vi "SP_Position_Set.vi"() -> ()   [LabVIEW 2013]
uses:
  <vilib>/event_ctls.llb/eventvkey.ctl
  Global_Not-Aus.vi
  <vilib>/Utility/file.llb/Write To Spreadsheet File (DBL).vi
  <vilib>/Utility/file.llb/Read From Spreadsheet File (string).vi
  Global_Start_Stop_Einzelschritt.vi
panel:
  in  "Stop Program":bool
  in  "Port for KOSY3":refnum<visa-resource-name>="COM2"
  in  "Port for Powersupply":refnum<visa-resource-name>="COM3"
  in  "Port for Write Head":refnum<visa-resource-name>="COM4"
  in  "Port for ED33":refnum<visa-resource-name>="COM7"
  in  "Port for ED32i":refnum<visa-resource-name>="COM8"
  in  "X,Y,Z Value Limits":T1={"mm Xmin "=0.0, "mm Xmax "=100.0, " mm Ymin "=0.0, "mm Ymax "=267.9, " mm Zmin"=0.0, "mm Zmax "=108.0, "Schritte oder mm Umin (0)"=0.0, "Schritte oder mm Umax (0)"=0.0, "Schritte oder mm Cmin (0)"=0.0, "Schritte oder mm Cmax (0)"=0.0, "Schritte oder mm Amin (0)"=0.0, "Schritte oder mm Amax (0)"=0.0, "Schritte oder mm Bmin (0)"=0.0, "Schritte oder mm Bmax (0)"=0.0}
  out "Error Out":errorcluster caption="error out"
  in  "Error In":errorcluster caption="error in"
  out "Movement":T2={"Axis"=36, "Direction(To/From)"=0, "Speed in mm/s\n (5)[0,025-20]"=5.0, "IV6"=FALSE} {"Direction(To/From)" items=["vom Endschalter weg", "zum Endschalter hin"]; "Speed in mm/s\n (5)[0,025-20]" min=0.025 max=20; "Axis" items=["X-Achse"=36, "Y-Achse"=37, "Z-Achse"=38, "U-Achse"=63]}
  out "Keyboard Press Display":cluster{"Speed(+/-)":i16, "Movement":T3}
  in  "Count":dbl
  in  "Move & Measure":bool
  in  "Clear Sensor Readings":bool
  in  "ED32i Active?":bool
  in  "ED33 Active?":bool
  out "ED33_output":string[][](array[string])
  out "ED32i_output":string[][](array[string])
  out "ED33":i32[](graph)
  out "ED32i":cluster{"Array 4[0]":i32, "Array 4[1]":i32}(graph)
  out "Steps":dbl
  out "Current Sequence":string[](array[string])
  in  "Clear Sequence":bool
  in  "Load Sequence":bool
  out "Sequence":string[][](array[string])
  in  "File  Select":path
  in  "Activate Sequence?":bool
  in  "Tab Control":enum32{"Page 2"}(tab)
  in  "Main Tab":enum32{"Page 1", "Page 2"}(tab)
  in  "Multiple Control":enum32{"Manual Control"}(tab)
  out "P6":dbl[](array[numeric])
  out "P5":dbl[](array[numeric])
  out "P4":dbl[](array[numeric])
  out "P3":dbl[](array[numeric])
  out "P7":dbl[](array[numeric])
  out "P2":dbl[](array[numeric])
  out "P1":dbl[](array[numeric])
  out "P8":dbl[](array[numeric])
  out "P9":dbl[](array[numeric])
  out "P10":dbl[](array[numeric])
  in  "Z axis":enum16{"Up", "Down"}(ring)
  in  "Y axis":enum16{"Forward", "Backward"}(ring)
  in  "X axis":enum16{"Left", "Right"}(ring)
  in  "Move Steps":bool
  in  "Steps(mm)":dbl[](array[numeric]) min=0.0
  in  "Go To":bool
  in  "Position":T4(ring)
  in  "Save":bool
  in  "Reset All":bool
  in  "Reset":bool
  in  "Import":bool
  in  "Export":bool
  in  "File Path":path=path "Y:/01_Projekte/EPN93031_Schreibplatz/8_Konstruktionsunterlagen/8.5_Software/COPY_KOSY Steuerung LabVIEW/1.New_Code_2014_2015/2Pole_strip_Position.txt"
  out "Speed":dbl(knob) scale=0.0..10.0
  out "Operation Done":string="Initialise"
  out "Current Status":string="Initialise"
  out "Moving":bool
  out "Stopped":bool
  in  "Home Position":bool
  out "Current Cordinates":T5 {"Schritte B" format="%#.4g"; "Schritte A" format="%#.4g"; "Schritte C" format="%#.4g"; "Schritte U" format="%#.4g"; "Z axis" format="%#.4g"; "Y axis" format="%#.4g"; "X axis" format="%#.4g"}
  # "Com port info"
  # "Instructions\n                                              Manual Control\n1. Run the program.\n2. Select 'Initialise' to start the program from first \n     or 'Continue' to continue the ongoing process.\n3. Select 'Normal Operation'.\n\nPolestrip Positions\n1. If already positions are already saved, select the corresponding \n    file in 'File Path' and then click 'Import' to get the corresponding\n    positions displayed on the front panel. \n2. Set the 'Speed' using (+/-) for the movement.\n3. Select a position from the dropdown 'Position'and click 'Go To'.\n    Else, \n1. Set the 'Speed' using (+/-) for the movement.\n2. Set the length for movement in 'Steps(mm)'  in corresponding \n    axis and also the direction of travel in the selected axis. \n    Then press 'Move'.\n3. Once desired position is reached, select a position from the \n    dropdown 'Position' and click 'Save'.\n4. Once all positions are saved in front panel, select the file  to be \n     saved in 'File Path' and click 'Export' to save positions to a text file.\n5. Select a position from the dropdown 'Position' and \n    Click 'Reset' to clear individual position.\n6. Click 'Reset All' to clear all positions.\n \nSensor Readings\nContinuous measurement\n1.Activate the sensor to be read from 'Read Sensors' tab.\n2.Set the length for movement in 'Steps(mm)' in corresponding \n    axis and also the direction of travel in the selected axis. \n    Then press 'Move'.\nMove and Measure\n1. Activate the sensor to be read from 'Read Sensors' tab.\n2.Set 'Count' to the number of times to measure.\n2.Set the length for movement in 'Steps(mm)' in corresponding \n    axis and also the direction of travel in the selected axis. \n    Then press 'Move Measure'.\n\n1. Click 'Clear' in 'Read Sensors' tab to clear the sensor readings.\n\n                                          Automatic Execution\n1. Run the program.\n2. Select 'Initialise' to start the program from first \n     or 'Continue' to continue the ongoing process.\n3. Select 'Normal Operation'.\n4. Select the corresponding file in 'File Select' and then click 'Load' \n    to get the corresponding codes in 'Sequence' .\n5. Click 'Clear' to clear sequence.\n6. Click 'Activate Sequence?' to run the automatic execution. \n\n                                                       General\n1. Click 'Stop Program' to stop the running program.\n2. Click 'Home Position' to take the write head to (0,0,0)."
  # "Instructions\n\n1. Set the 'Speed' using (+/-) for the movement.\n2. Arrow keys can be used to move the platform in a particular\n    axis and corresponding direction.\n     First press - move / Second press - stop\n     OR,\n    Set the length for movement in 'Steps(mm)'  in corresponding \n    axis and also the direction of travel in the selected axis. \n    Then press 'Move'.\n3. Once desired position is reached, select a position from the \n    dropdown 'Position' and click 'Save'.\n4. Once all positions are saved in front panel, select the file  to be \n     saved, in 'File Path' and click 'Export' to save positions to a text file.\n5. Select a position from the dropdown 'Position' and \n    Click 'Reset' to clear individual position.\n6. Click 'Reset All' to clear all positions.\n7. Once positions are saved, select the file in 'File Path' and\n     then 'Import' to get the positions displayed ."
  # "Polestrip Positions"
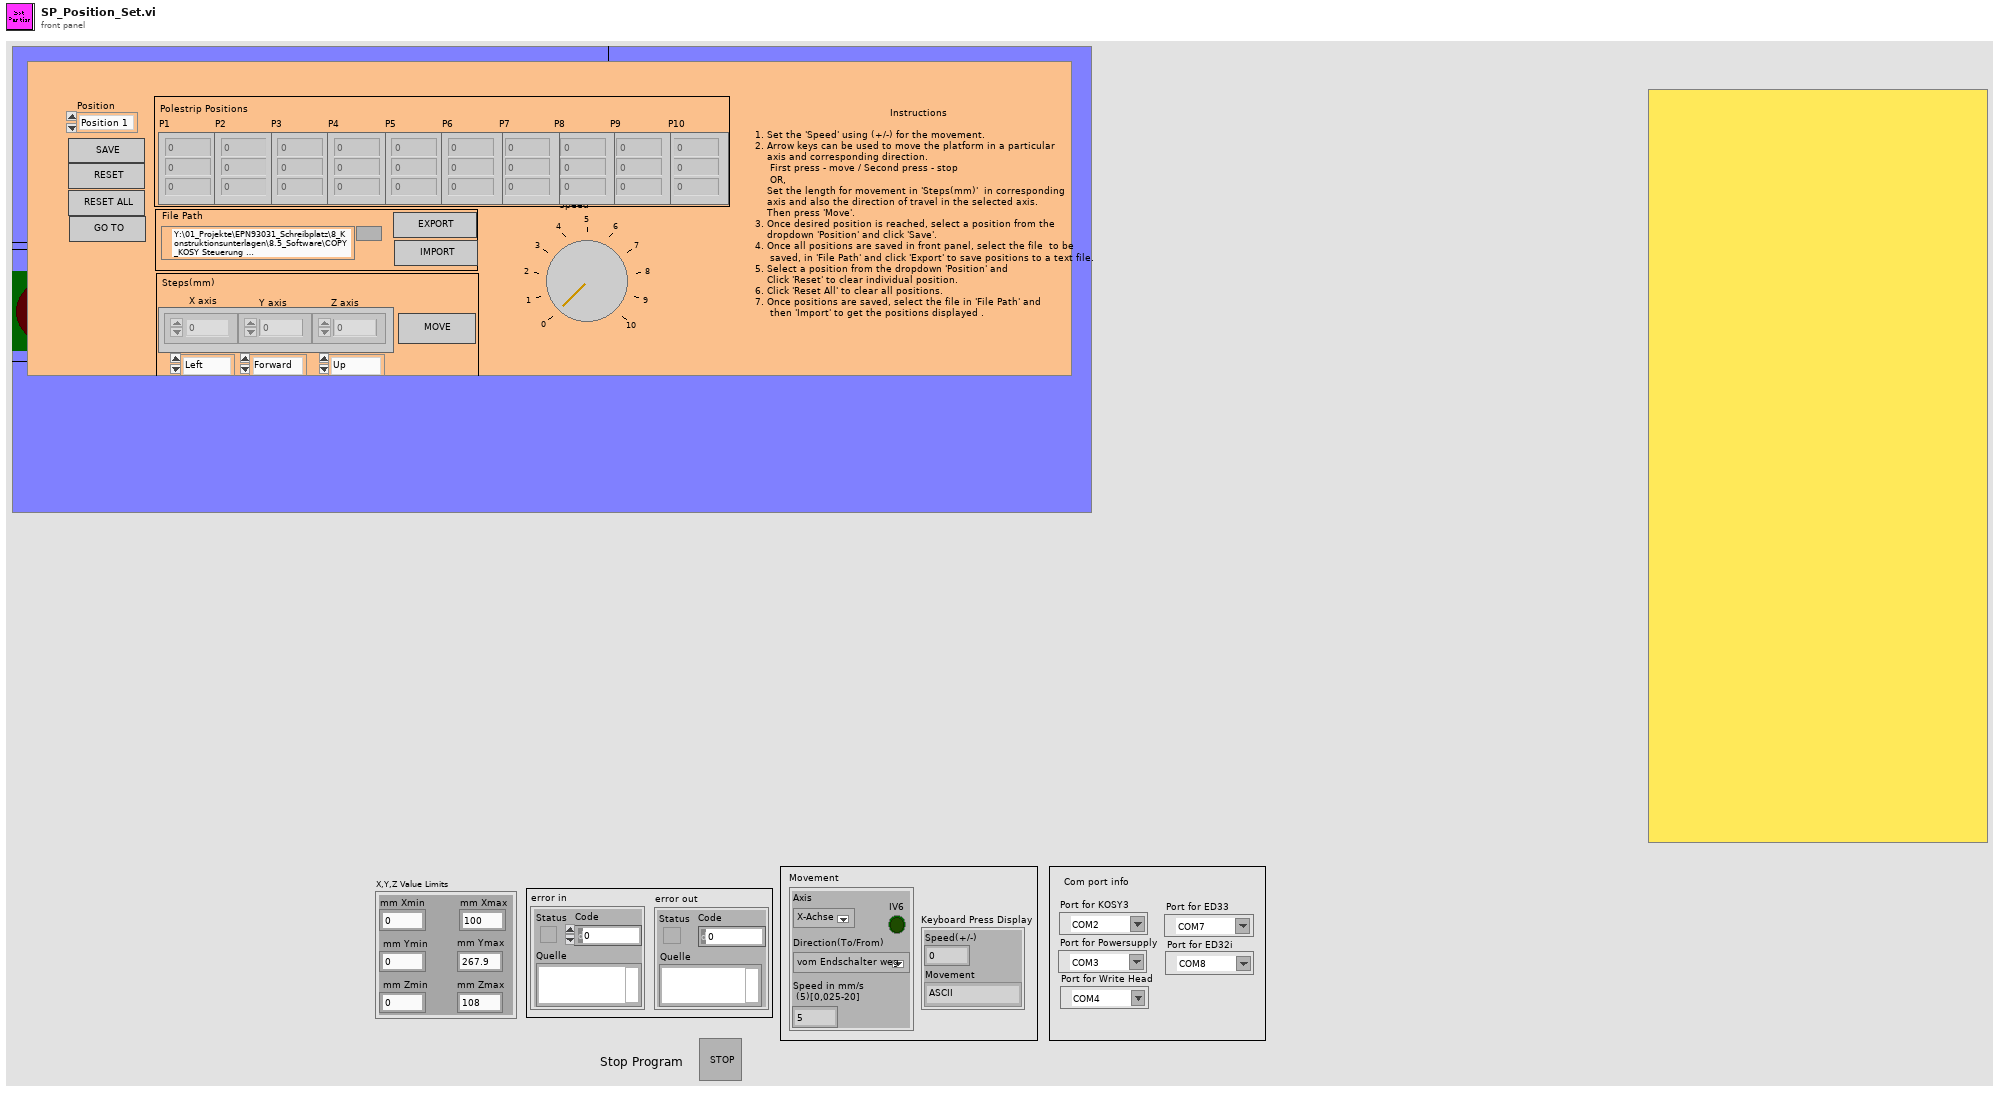
[diagram p1: front panel]
types:
  T1 = cluster{"mm Xmin ":sgl, "mm Xmax ":sgl, " mm Ymin ":sgl, "mm Ymax ":sgl, " mm Zmin":sgl, "mm Zmax ":sgl, "Schritte oder mm Umin (0)":sgl, "Schritte oder mm Umax (0)":sgl, "Schritte oder mm Cmin (0)":sgl, "Schritte oder mm Cmax (0)":sgl, "Schritte oder mm Amin (0)":sgl, "Schritte oder mm Amax (0)":sgl, "Schritte oder mm Bmin (0)":sgl, "Schritte oder mm Bmax (0)":sgl}
  T2 = cluster{"Axis":u8, "Direction(To/From)":u8, "Speed in mm/s\n (5)[0,025-20]":sgl, "IV6":bool}
  T3 = typedef "eventvkey.ctl" = enum16{"ASCII", "Enter", "Return", "Shift", "Ctrl", "Alt", "Cmd", "Opt", "Caps", "NumLock", "Clear", "Break", "Up", "Down", "Left", "Right", "Insert", "Delete", "Home", "End", "PageUp", "PageDown", "Escape", "Help", "Pause", "ScrollLock", "F1", "F2", "F3", "F4", "F5", "F6", "F7", "F8", "F9", "F10", "F11", "F12", "F13", "F14", "F15", "F16", "F17", "F18", "F19", "F20", "F21", "F22", "F23", "F24", "Play", "VolumeUp", "VolumeDown", "Mute", "Two Byte Char"}
  T4 = enum16{"Position 1", "Position 2", "Position 3", "Position 4", "Position 5", "Position 6", "Position 7", "Position 8", "Position 9", "Position 10"}
  T5 = cluster{"X axis":sgl, "Y axis":sgl, "Z axis":sgl, "Schritte U":sgl, "Schritte C":sgl, "Schritte A":sgl, "Schritte B":sgl}
  T6 = cluster{"Geschwindigkeit X in mm/s\n(5) [0,025-15]":sgl, "Geschwindigkeit Y in mm/s\n(5) [0,025-15]":sgl, "Geschwindigkeit Z in mm/s\n(5) [0,025-15]":sgl, "GeschwindigkeitU in mm/s\n(5) [0,025-15]":sgl}
  T7 = cluster{"Schritte X":sgl, "Schritte Y":sgl, "Schritte Z":sgl, "Schritte U":sgl, "Schritte C":sgl, "Schritte A":sgl, "Schritte B":sgl}
  T8 = cluster{"[0]":dbl, "[1]":dbl, "[2]":dbl, "[3]":dbl, "[4]":dbl, "[5]":dbl, "[6]":dbl, "[7]":dbl, "[8]":dbl}
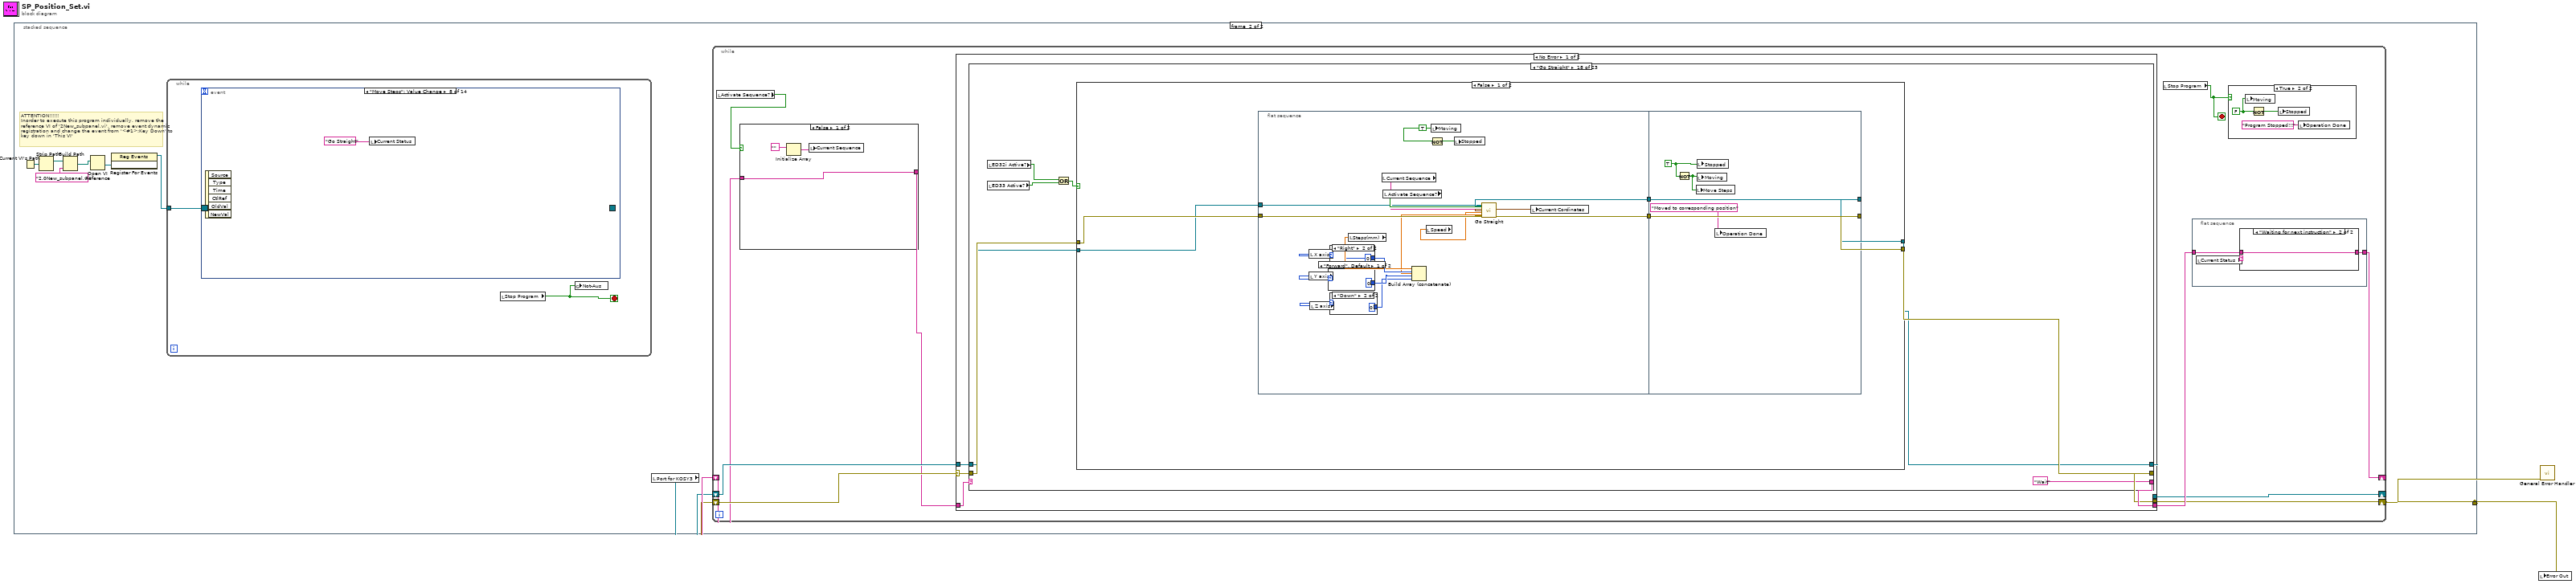
[diagram p0: block diagram]
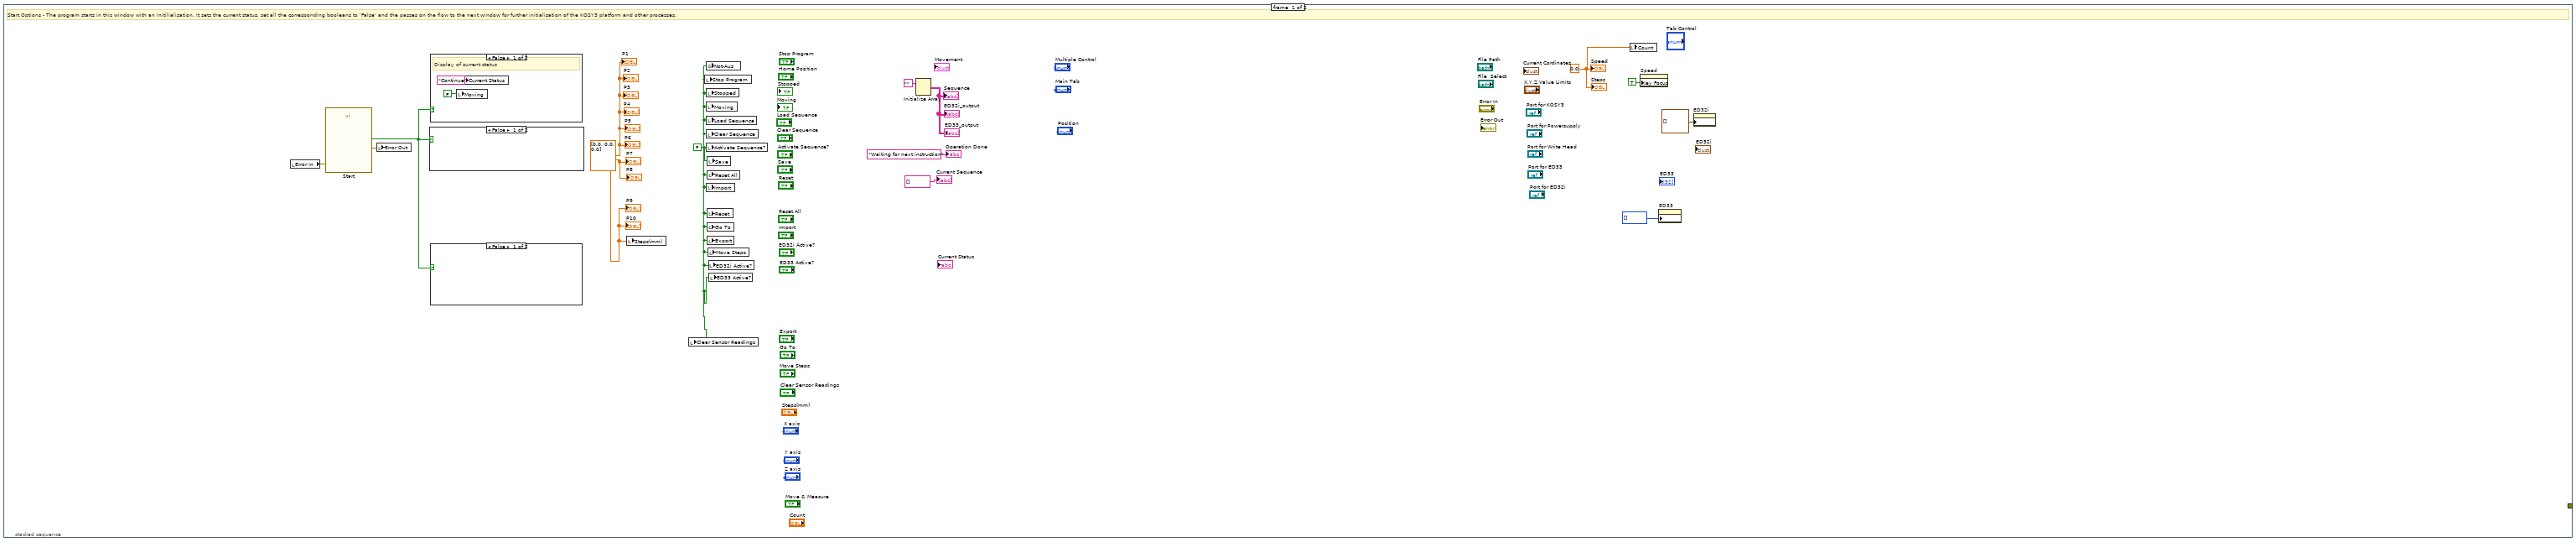
[diagram p2: hidden frame]
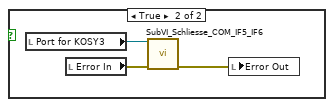
[diagram p3: hidden frame]
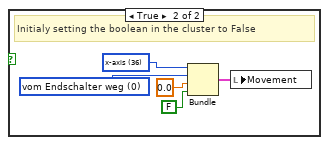
[diagram p4: hidden frame]
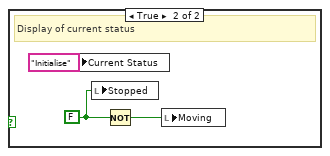
[diagram p5: hidden frame]
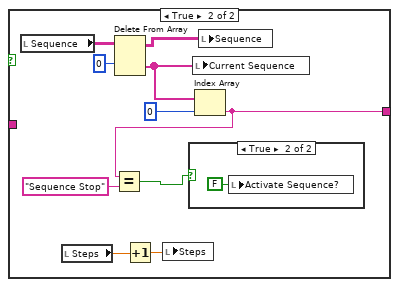
[diagram p6: hidden frame]
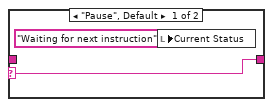
[diagram p9: hidden frame]
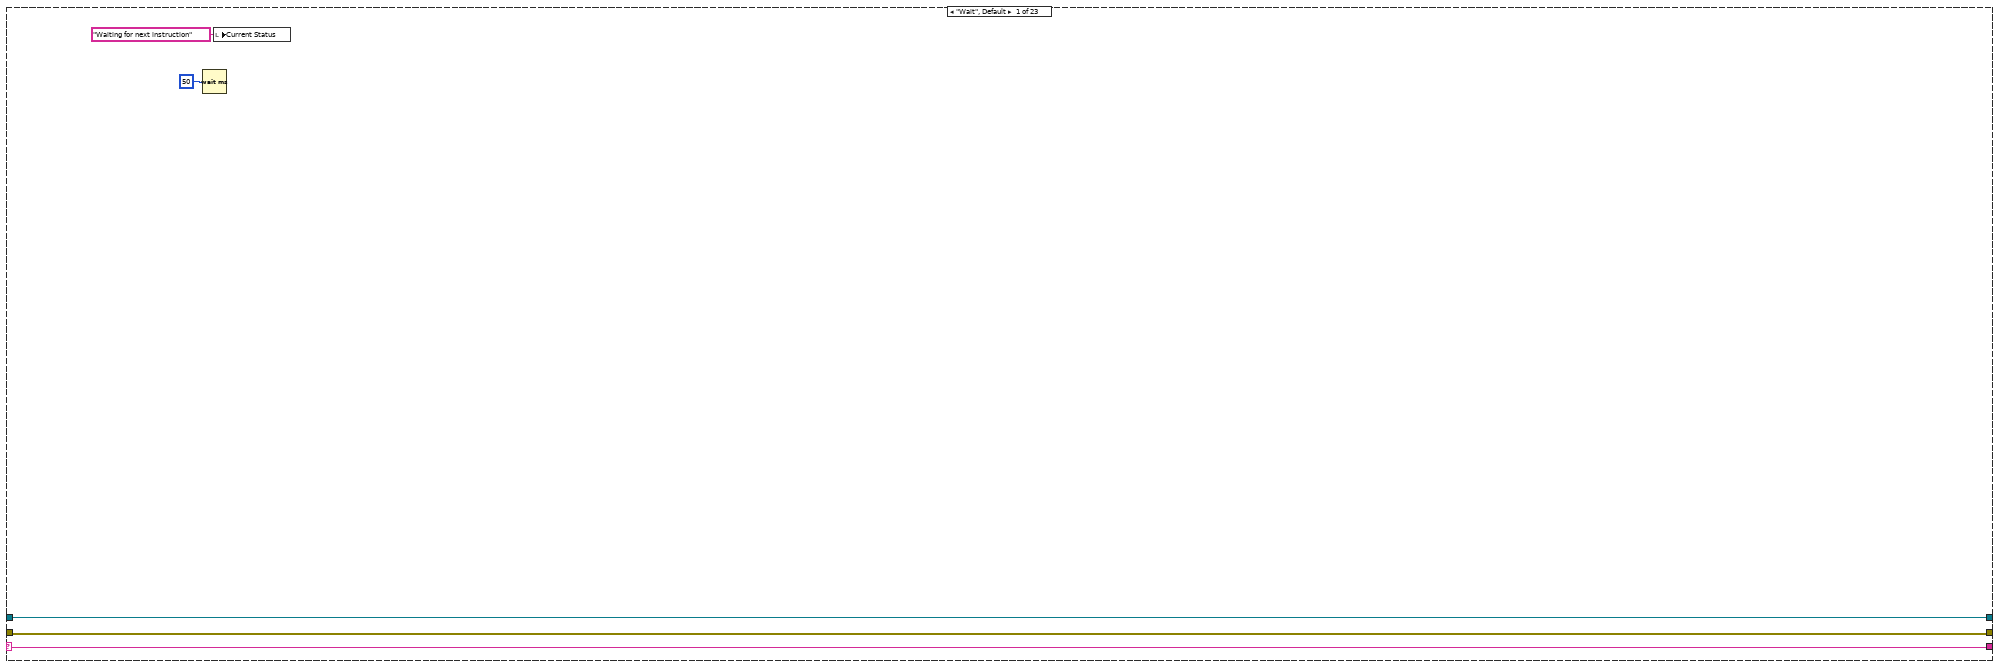
[diagram p10: hidden frame]
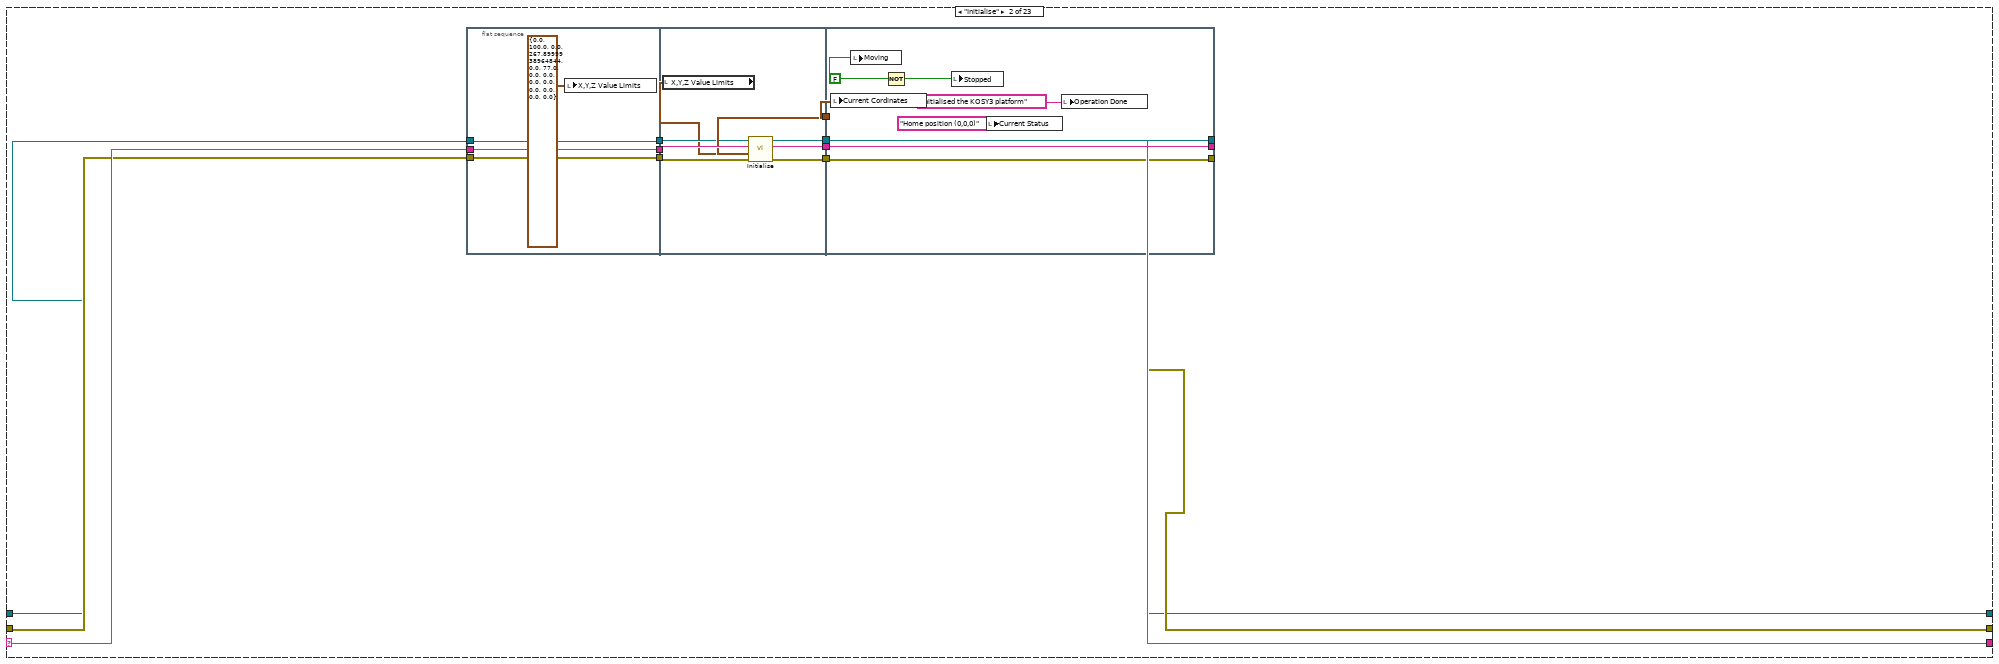
[diagram p11: hidden frame]
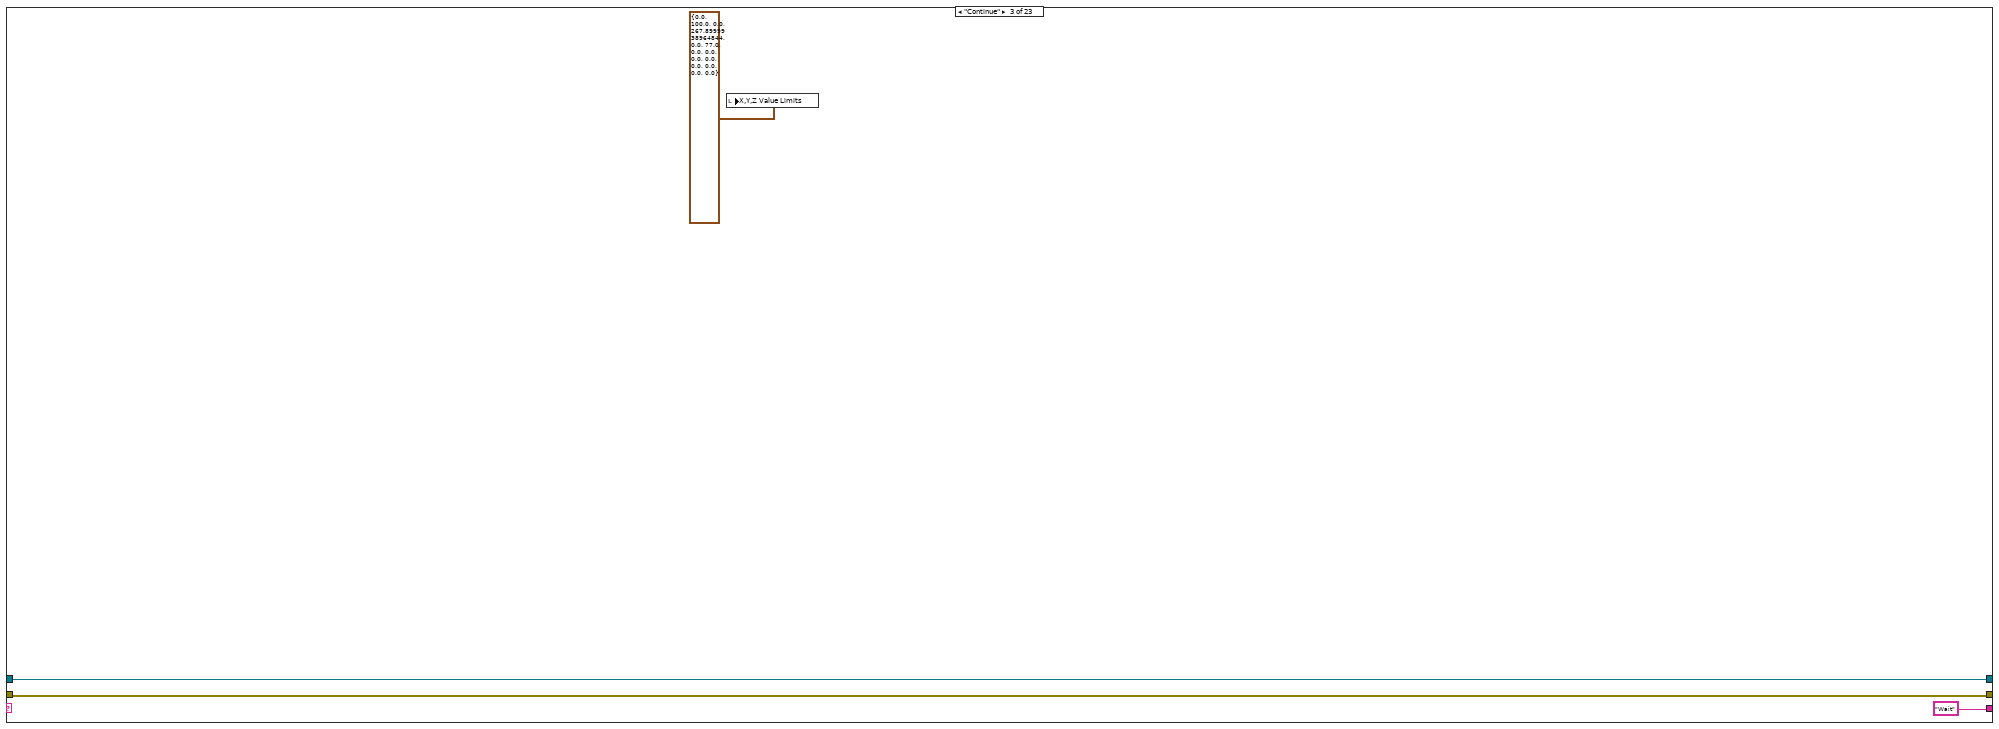
[diagram p12: hidden frame]
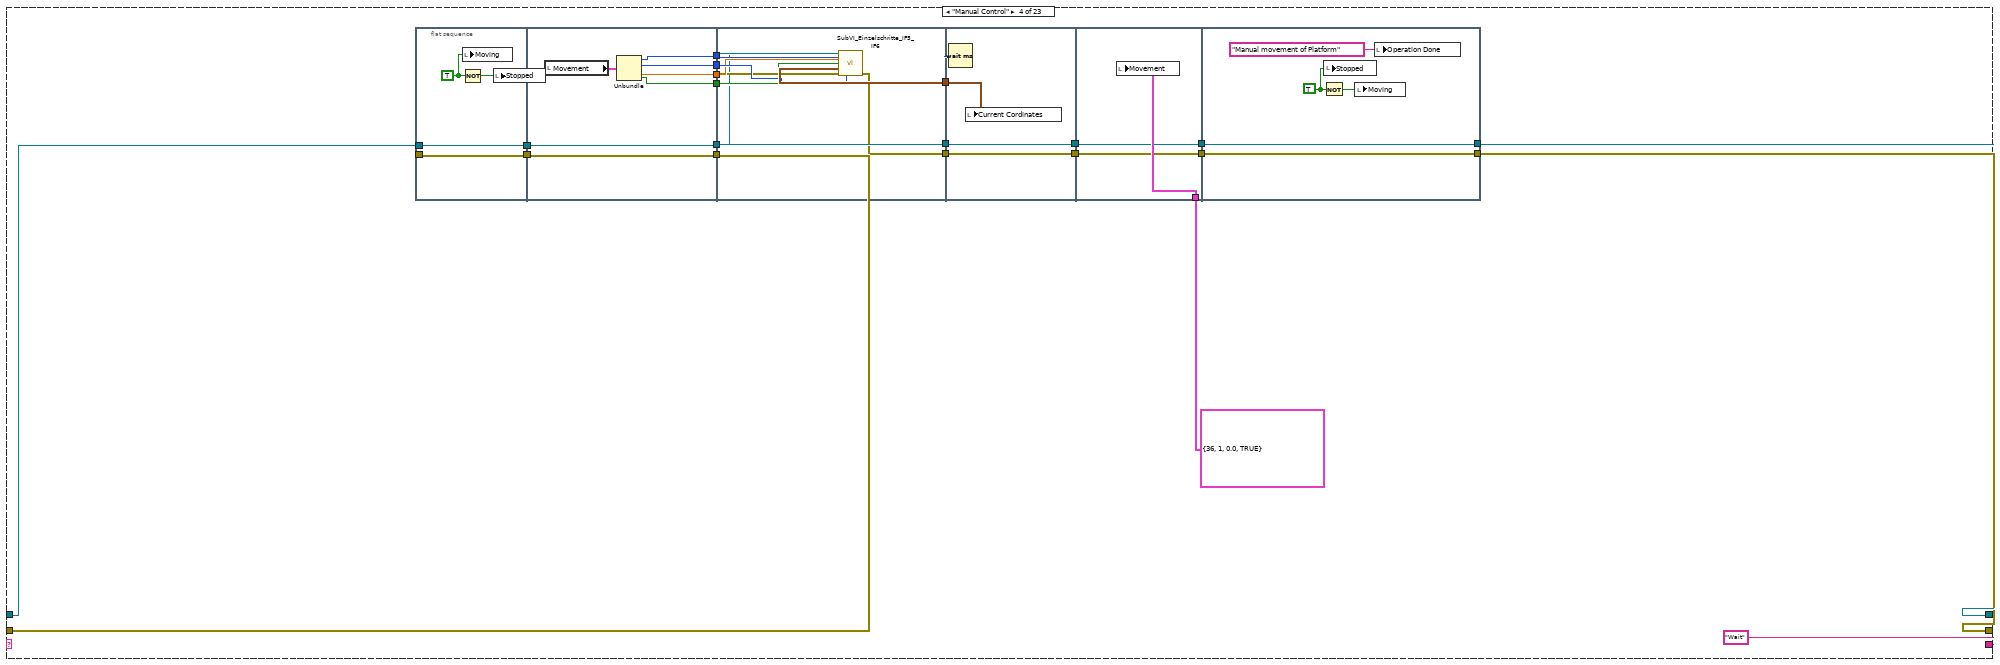
[diagram p13: hidden frame]
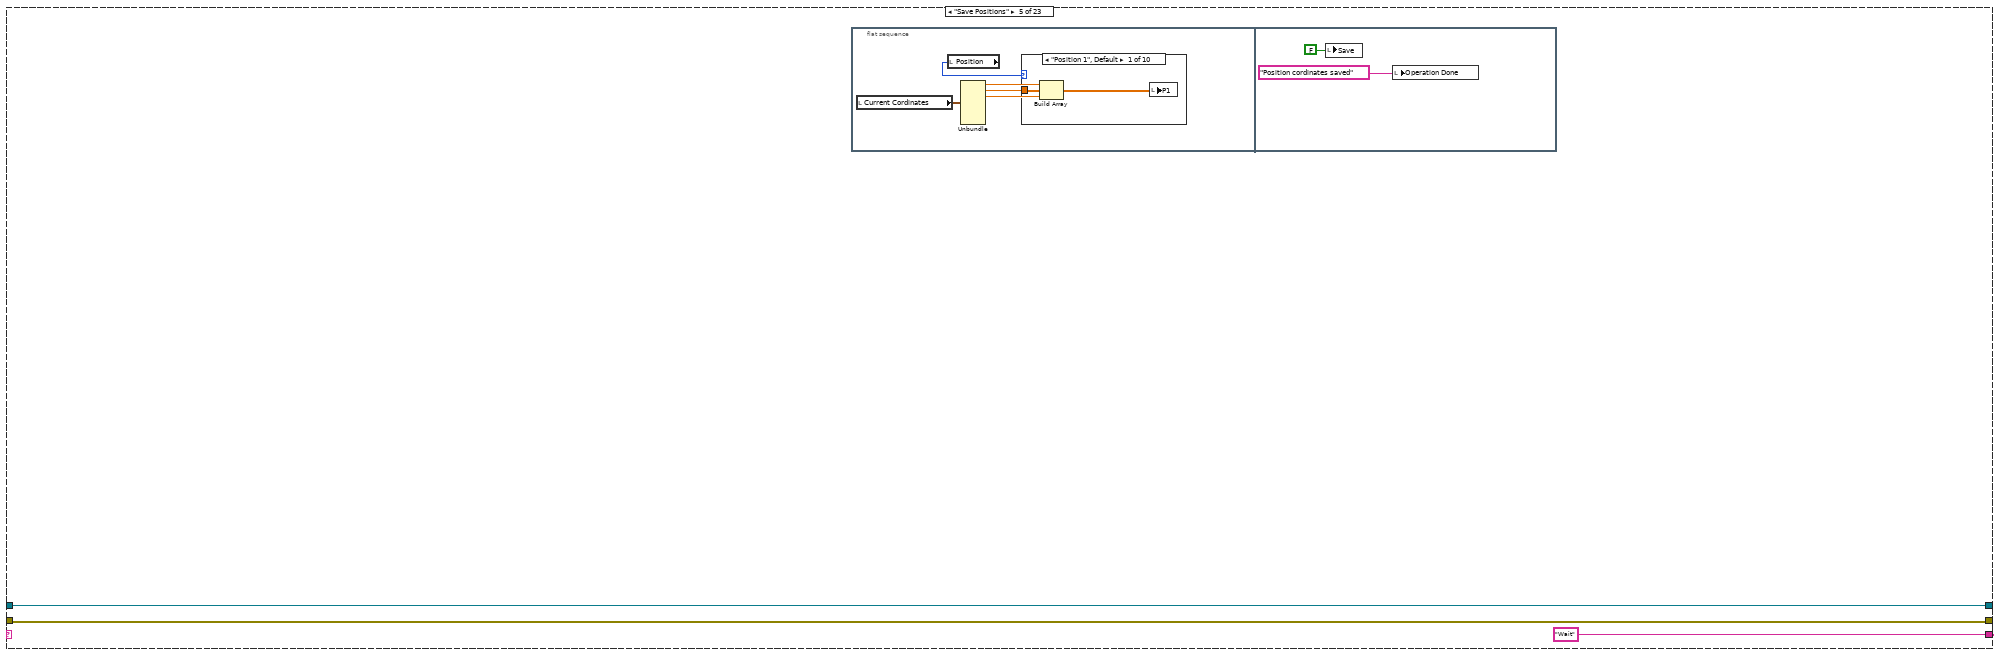
[diagram p14: hidden frame]
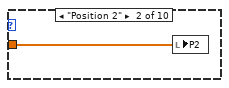
[diagram p15: hidden frame]
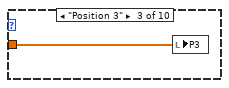
[diagram p16: hidden frame]
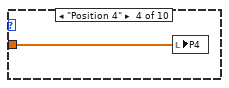
[diagram p17: hidden frame]
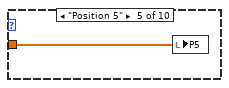
[diagram p18: hidden frame]
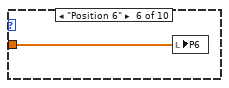
[diagram p19: hidden frame]
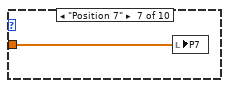
[diagram p20: hidden frame]
diagram:
  n1 = stacked-sequence {
    tunnel: [_ w34] -> w1
    frame #0 {
      w3 = 0.0 ("Speed")
      w4 = dbl[] [0.0, 0.0, 0.0] ("P1")
      w7 = FALSE ("Moving")
      # "Start Options - The program starts in this window with an initilialisation. It sets the current status, set all the corresponding booleans to 'False' and the passes on the flow to the next window for further initialisation of the KOSY3 platform and other processes."
      n2 = local read "Error In"() -> (w14:errorcluster)
      n3 = call "Start"("error in (no error)"=w14) -> ("Initialise"=w12:bool, "error out"=w13:errorcluster)  [unwired: 17 in]
      n4 = local write "Error Out"(w13) -> ()
      n5 = case shown="False" w12 {
        frame False {
        }
        frame True {
          n6 = local read "Port for KOSY3"() -> (w17:refnum<visa-resource-name>)
          n7 = local read "Error In"() -> (w16:errorcluster)
          n8 = call "SubVI_Schliesse_COM_IF5_IF6.vi"("VISA resource name in"=w17, "error in"=w16) -> ("error out"=w15:errorcluster)  [unwired: 13 in]
          n9 = local write "Error Out"(w15) -> ()
        }
      }
      n10 = case shown="False" w12 {
        frame False {
          # "Display of current status"
          n11 = local write "Moving"(FALSE ("Stopped")) -> ()
          n12 = local write "Current Status"("Continue") -> ()
        }
        frame True {
          w25 = FALSE ("Stopped")
          # "Display of current status"
          n13 = local write "Current Status"("Initialise") -> ()
          n14 = local write "Stopped"(w25) -> ()
          n15 = Not(x=w25) -> (.not. x?=w26:bool)
          n16 = local write "Moving"(w26) -> ()
        }
      }
      n17 = case shown="False" w12 {
        frame False {
        }
        frame True {
          w21 = u16 0 items=["vom Endschalter weg", "zum Endschalter hin"]
          w22 = u16 36 items=["x-axis"=36, "y-axis"=37, "z-axis"=38]
          # "Initialy setting the boolean in the cluster to False"
          n18 = Bundle(w22, w21, 0.0, FALSE) -> (w18:cluster{u16, u16, dbl, bool})  [unwired: 1 in]
          n19 = local write "Movement"(w18) -> ()
        }
      }
      n20 = local write "Steps(mm)"(w4) -> ()
      n21 = local write "Clear Sensor Readings"(w7) -> ()
      n22 = local write "Stop Program"(w7) -> ()
      n23 = global write "Global_Not-Aus.vi" "Not-Aus"(w7) -> ()
      n24 = local write "Stopped"(w7) -> ()
      n25 = local write "Moving"(w7) -> ()
      n26 = local write "Load Sequence"(w7) -> ()
      n27 = local write "Clear Sequence"(w7) -> ()
      n28 = local write "Activate Sequence?"(w7) -> ()
      n29 = local write "Import"(w7) -> ()
      n30 = local write "Reset All"(w7) -> ()
      n31 = local write "Reset"(w7) -> ()
      n32 = local write "Go To"(w7) -> ()
      n33 = local write "Export"(w7) -> ()
      n34 = local write "Save"(w7) -> ()
      n35 = local write "Move Steps"(w7) -> ()
      n36 = local write "ED32i Active?"(w7) -> ()
      n37 = local write "ED33 Active?"(w7) -> ()
      n38 = Initialize Array("" ("element")) -> (→"Sequence" →"ED32i_output" →"ED33_output":string[][])  [unwired: 2 in]
      n39 = local write "Count"(w3) -> ()
      n40 = property on="Speed" class="Knob (strict)"("Key Focus"=TRUE) -> ()  [unwired: 2 in, 2 out]
      n41 = property on="ED33" class="WFChart (strict)"("History Data"=i32[] []) -> ()  [unwired: 2 in, 2 out]
      n42 = property on="ED32i" class="WFChart (strict)"("History Data"=cluster{"Array 4[0]":i32, "Array 4[1]":i32}[] []) -> ()  [unwired: 2 in, 2 out]
      "Speed" <- w3
      "P1" <- w4
      "P2" <- w4
      "P3" <- w4
      "P7" <- w4
      "P4" <- w4
      "P5" <- w4
      "P6" <- w4
      "P8" <- w4
      "P9" <- w4
      "P10" <- w4
      "Current Sequence" <- string[] [] ("Current Sequence")
      "Operation Done" <- "Waiting for next instruction" ("Operation Done")
      "Steps" <- w3
    }
    frame #1 {
      # "ATTENTION!!!!!!\nInorder to execute this program individually, remove the reference VI of '2New_subpanel.vi', remove event dynamic registration and change the event from '<#1>:Key Down' to key down in 'This VI'"
      n43 = Current VI's Path() -> (path=w32:path)
      n44 = Strip Path(path=w32) -> (stripped path=w31:path)  [unwired: 1 out]
      n45 = Build Path(base path=w31, name or relative path="2.0New_subpanel.vi") -> (appended path=w29:path)
      n46 = Open VI Reference(vi path=w29) -> (vi reference=w33:refnum<vi>)  [unwired: 5 in, 1 out]
      n47 = register-events(w33) -> (reference out=w28:refnum<event-registration>)  [unwired: 2 in, 1 out]
      n48 = while {
        tunnel: w28 -> [w692]
        stop <- w691 stop-if-true
        n49 = event shown="[7] \"Move Steps\": Value Change" {
          selector: w692 -> [_ w694 _ _ _ _ _ _ _ _ _ _ _ _]
          dyn-events: [_ w694 _ _ _ _ _ _ _ _ _ _ _ _] -> _
          timeout: _ -> [_ _ _ _ _ _ _ _ _ _ _ _ _ _]
          event Timeout {
            n50 = event-data() -> ()  [unwired: 1 in, 2 out]
            n51 = global write "Global_Start_Stop_Einzelschritt.vi" "Boolesch"(FALSE ("Boolesch")) -> ()
          }
          event Key Down {
            # "This window checks for the key press in key board. Upon detection, it would set speed and (or) movement cluster and also updates the status."
            n52 = event-data() -> ("Char"=w695:i16, "VKey"=w697:T3)  [unwired: 1 in, 8 out]
            n53 = Wait (ms)(milliseconds to wait=u32 200) -> ()  [unwired: 1 out]
            n54 = Bundle("Char"=w695, "VKey"=w697) -> (→"Keyboard Press Display":cluster{"Char":i16, "VKey":T3})  [unwired: 1 in]
            n55 = local read "Moving"() -> (w699:bool)
            n56 = case shown="False" w699 {
              tunnel: w697 -> [w705 _]
              tunnel: w695 -> [w707 _]
              frame False {
                n57 = case shown="\"Up\"" w705 {
                  tunnel: [w708 w711 w714 w717 w720 w723 FALSE] -> w704
                  tunnel: [w710 w713 w716 w719 w722 w725 _] -> w702
                  tunnel: [w709 w712 w715 w718 w721 w724 _] -> w701
                  tunnel: TRUE -> [w708 w711 w714 w717 w720 w723 _]
                  frame "Left" {
                    w709 = u16 1 items=["vom Endschalter weg", "zum Endschalter hin"]
                    w710 = u16 36 items=["x-axis"=36, "y-axis"=37, "z-axis"=38]
                    # "Direction control(VKey identifies the directional keys)"
                  }
                  frame "Right" {
                    w712 = u16 0 items=["vom Endschalter weg", "zum Endschalter hin"]
                    w713 = u16 36 items=["x-axis"=36, "y-axis"=37, "z-axis"=38]
                    # "Direction control"
                  }
                  frame "Up" {
                    w715 = u16 1 items=["vom Endschalter weg", "zum Endschalter hin"]
                    w716 = u16 37 items=["x-axis"=36, "y-axis"=37, "z-axis"=38]
                    # "Direction control"
                  }
                  frame "Down" {
                    w718 = u16 0 items=["vom Endschalter weg", "zum Endschalter hin"]
                    w719 = u16 37 items=["x-axis"=36, "y-axis"=37, "z-axis"=38]
                  }
                  frame "PageUp" {
                    w721 = u16 1 items=["vom Endschalter weg", "zum Endschalter hin"]
                    w722 = u16 38 items=["x-axis"=36, "y-axis"=37, "z-axis"=38]
                  }
                  frame "PageDown" {
                    w724 = u16 0 items=["vom Endschalter weg", "zum Endschalter hin"]
                    w725 = u16 38 items=["x-axis"=36, "y-axis"=37, "z-axis"=38]
                  }
                  frame "Return", Default {
                  }
                }
                n58 = local read "Speed"() -> (w700:dbl)
                n59 = call "Speed_set.vi"("Speed"=w700, "Char"=w707) -> ("Speed"=w706:dbl)
                n60 = local write "Speed"(w706) -> ()
                n61 = case shown="True" w704 {
                  tunnel: w706 -> [_ w730]
                  tunnel: w702 -> [_ w729]
                  tunnel: w701 -> [_ w728]
                  frame False {
                  }
                  frame True {
                    n62 = Bundle(w729, w728, "Speed"=w730, TRUE) -> (w727:cluster{u16, u16, "Speed":dbl, bool})  [unwired: 1 in]
                    n63 = local write "Movement"(w727) -> ()
                    n64 = local write "Current Status"("Manual Control" ("Status")) -> ()
                  }
                }
              }
              frame True {
                n65 = global write "Global_Start_Stop_Einzelschritt.vi" "Boolesch"(TRUE) -> ()
                n66 = local write "Moving"(FALSE) -> ()
              }
            }
          }
          event "Home Position": Value Change {
            # "This window corresponds to the 'Home position' button on the Front Panel. Pressing the button will take KOSY3 paltform to the home position (0,0,0)"
            n67 = event-data() -> ()  [unwired: 1 in, 6 out]
            n68 = local write "Current Status"("Home Position" ("Status")) -> ()
          }
          event "Save": Value Change {
            # "When the 'SAVE' button in the Front Panel is pressed, it would save the current cordinates of the KOSY3 platform to the selected position."
            n69 = event-data() -> ()  [unwired: 1 in, 6 out]
            n70 = local write "Current Status"("Save Positions" ("Status")) -> ()
          }
          event "Reset": Value Change {
            # "When 'RESET' in the Front Panel is pressed, it resets the cordinates in the selected position to (0,0,0)"
            n71 = event-data() -> ()  [unwired: 1 in, 6 out]
            n72 = local write "Current Status"("Reset Position" ("Status")) -> ()
          }
          event "Reset All": Value Change {
            # "When 'RESET ALL' in the Front Panel is pressed, it resets the cordinates in all positions to (0,0,0)"
            n73 = event-data() -> ()  [unwired: 1 in, 6 out]
            n74 = local write "Current Status"("Reset All" ("Status")) -> ()
          }
          event "Go To": Value Change {
            n75 = event-data() -> ()  [unwired: 1 in, 6 out]
            n76 = local write "Current Status"("Go Position" ("Status")) -> ()
          }
          event "Move Steps": Value Change {
            n77 = event-data() -> ()  [unwired: 1 in, 6 out]
            n78 = local write "Current Status"("Go Straight" ("Status")) -> ()
          }
          event "Move & Measure": Value Change {
            n79 = event-data() -> ()  [unwired: 1 in, 6 out]
            n80 = local write "Current Status"("Move & Measure" ("Status")) -> ()
          }
          event "Import": Value Change {
            n81 = event-data() -> ()  [unwired: 1 in, 6 out]
            n82 = local write "Current Status"("Import Cordinates" ("Status")) -> ()
          }
          event "Export": Value Change {
            n83 = event-data() -> ()  [unwired: 1 in, 6 out]
            n84 = local write "Current Status"("Export Cordinates" ("Status")) -> ()
          }
          event "Load Sequence": Value Change {
            n85 = event-data() -> ()  [unwired: 1 in, 6 out]
            n86 = local write "Current Status"("Load Sequence" ("Status")) -> ()
          }
          event "Clear Sequence": Value Change {
            n87 = event-data() -> ()  [unwired: 1 in, 6 out]
            n88 = local write "Current Status"("Clear Sequence" ("Status")) -> ()
          }
          event "Clear Sensor Readings": Value Change {
            n89 = event-data() -> ()  [unwired: 1 in, 6 out]
            n90 = local write "Current Status"("Clear SensorReadings" ("Status")) -> ()
          }
        }
        n91 = local read "Stop Program"() -> (w691:bool)
        n92 = global write "Global_Not-Aus.vi" "Not-Aus"(w691) -> ()
      }
      n93 = local read "Port for KOSY3"() -> (w35:refnum<visa-resource-name>)
      n94 = local read "Current Status"() -> (w37:string)
      n95 = local read "Error In"() -> (w36:errorcluster)
      n96 = while {
        shift-right: [w42] -> w34
        shift-left: w36 -> [w47]
        shift-right: [w43] -> _
        shift-left: w35 -> [w44]
        shift-right: [w45] -> _
        shift-left: w37 -> [w41]
        stop <- w38 stop-if-true
        n97 = local read "Activate Sequence?"() -> (w39:bool)
        n98 = case shown="False" w39 {
          tunnel: w41 -> [w50 _]
          tunnel: [w50 w55] -> w40
          frame False {
            n99 = Initialize Array("") -> (w48:string[])  [unwired: 1 in]
            n100 = local write "Current Sequence"(w48) -> ()
          }
          frame True {
            n101 = local read "Sequence"() -> (w60:string[][])
            n102 = local read "Steps"() -> (w52:dbl)
            n103 = Delete From Array(array=w60, index (row)=0) -> (deleted portion=w57:string[], array with subset deleted=w58:string[][])  [unwired: 2 in]
            n104 = Increment(x=w52) -> (x+1=w51:dbl)
            n105 = local write "Steps"(w51) -> ()
            n106 = local write "Current Sequence"(w57) -> ()
            n107 = Index Array(array=w57, index=0) -> (element=w55:string)
            n108 = Equal?(x=w55, y="Sequence Stop") -> (x = y?=w53:bool)
            n109 = case shown="True" w53 {
              frame False {
              }
              frame True {
                n110 = local write "Activate Sequence?"(FALSE ("Activate Sequence?")) -> ()
              }
            }
            n111 = local write "Sequence"(w58) -> ()
          }
        }
        n112 = case shown="No Error" w47 {
          selector: w47 -> [w73 w686]
          tunnel: w40 -> [w76 _]
          tunnel: [w75 "Error" ("String 2")] -> w46
          tunnel: w44 -> [w74 w687]
          tunnel: [w71 w687] -> w43
          tunnel: [w72 w686] -> w42
          frame No Error {
            n113 = case shown="\"Go Straight\"" w76 {
              selector: w76 -> [w80 w94 _ _ _ _ _ _ _ _ _ _ _ _ _ _ _ _ _ _ _ _ _]
              tunnel: [w80 w91 "Wait" ("String 2") "Wait" "Wait" ("String 2") "Wait" ("String 2") "Wait" ("String 2") "Wait" ("String 2") "Wait" ("String 2") "Wait" ("String 2") "Wait" ("String 2") "Wait" ("String 2") "Wait" ("String 2") "Wait" ("String 2") "Wait" ("String 2") "Wait" ("String 2") "Wait" ("String 2") "Wait" ("String 2") "Wait" ("String 2") "Wait" ("String 2") "Wait" ("String 2") "Wait" ("String 2") "Wait" ("String 2")] -> w75
              tunnel: w74 -> [w77 w89 w117 w127 w173 w194 w211 w221 w253 w269 w308 w331 w338 w347 w356 w365 w379 w414 w536 w565 w573 w671 w678]
              tunnel: w73 -> [w78 w90 w115 w130 w172 w193 w210 w220 w254 w270 w310 w332 w339 w346 w357 w364 w380 w415 w534 w564 w574 w670 w680]
              tunnel: [w78 w87 w115 w122 w172 w193 w210 w218 w254 w270 w305 w332 w339 w346 w357 w364 w381 w413 w534 w564 w574 w670 w679] -> w72
              tunnel: [w77 w85 w117 w126 w173 w194 w211 w219 w253 w269 w307 w331 w338 w347 w356 w365 w382 w412 w536 w565 w572 w671 w678] -> w71
              frame "Wait", Default {
                n114 = Wait (ms)(milliseconds to wait=50) -> ()  [unwired: 1 out]
                n115 = local write "Current Status"("Waiting for next instruction" ("Status")) -> ()
              }
              frame "Initialise" {
                n116 = flat-sequence {
                  tunnel: w89 -> [w96]
                  tunnel: w90 -> [w97]
                  tunnel: w94 -> [w98]
                  tunnel: [w98] -> w84
                  tunnel: [w97] -> w83
                  tunnel: [w96] -> w82
                  tunnel: [w105] -> w93
                  tunnel: [w104] -> w92
                  tunnel: [w101] -> w88
                  tunnel: [w100] -> w86
                  tunnel: w84 -> [w106]
                  tunnel: w83 -> [w103]
                  tunnel: w82 -> [w102]
                  tunnel: w93 -> [w111]
                  tunnel: w92 -> [w110]
                  tunnel: [w110] -> w91
                  tunnel: [w108] -> w85
                  tunnel: w88 -> [w108]
                  tunnel: [w107] -> w87
                  tunnel: w86 -> [w107]
                  frame #0 {
                    n117 = local write "X,Y,Z Value Limits"(T1 {"mm Xmin "=0.0, "mm Xmax "=100.0, " mm Ymin "=0.0, "mm Ymax "=267.9, " mm Zmin"=0.0, "mm Zmax "=77.0, "Schritte oder mm Umin (0)"=0.0, "Schritte oder mm Umax (0)"=0.0, "Schritte oder mm Cmin (0)"=0.0, "Schritte oder mm Cmax (0)"=0.0, "Schritte oder mm Amin (0)"=0.0, "Schritte oder mm Amax (0)"=0.0, "Schritte oder mm Bmin (0)"=0.0, "Schritte oder mm Bmax (0)"=0.0} ("X,Y,Z Value Limits")) -> ()
                  }
                  frame #1 {
                    n118 = local read "X,Y,Z Value Limits"() -> (w99:T1)
                    n119 = call "Initialise.vi"("error IO"=w103, "X,Y,Z values"=w99, "String"=w106, "Port for KOSY3"=w102) -> ("Fehler (Ausgang)"=w100:errorcluster, "Cordinates of the  KOSY3 Platform"=w105:T7, "String 2"=w104:string, "VISA-Referenz (Ausgang)"=w101:refnum<visa-resource-name>)
                  }
                  frame #2 {
                    w112 = FALSE ("Stopped")
                    n120 = local write "Current Cordinates"(w111) -> ()
                    n121 = local write "Moving"(w112) -> ()
                    n122 = Not(x=w112) -> (.not. x?=w113:bool)
                    n123 = local write "Stopped"(w113) -> ()
                    n124 = local write "Current Status"("Home position (0,0,0)" ("Status")) -> ()
                    n125 = local write "Operation Done"("Initialised the KOSY3 platform" ("Operation Done")) -> ()
                  }
                }
              }
              frame "Continue" {
                n126 = local write "X,Y,Z Value Limits"(T1 {"mm Xmin "=0.0, "mm Xmax "=100.0, " mm Ymin "=0.0, "mm Ymax "=267.9, " mm Zmin"=0.0, "mm Zmax "=77.0, "Schritte oder mm Umin (0)"=0.0, "Schritte oder mm Umax (0)"=0.0, "Schritte oder mm Cmin (0)"=0.0, "Schritte oder mm Cmax (0)"=0.0, "Schritte oder mm Amin (0)"=0.0, "Schritte oder mm Amax (0)"=0.0, "Schritte oder mm Bmin (0)"=0.0, "Schritte oder mm Bmax (0)"=0.0} ("X,Y,Z Value Limits")) -> ()
              }
              frame "Manual Control" {
                n127 = flat-sequence {
                  tunnel: [w141] -> w131
                  tunnel: w130 -> [w141]
                  tunnel: [w140] -> w128
                  tunnel: w127 -> [w140]
                  tunnel: [w149] -> w138
                  tunnel: [w148] -> w137
                  tunnel: [w147] -> w136
                  tunnel: [w146] -> w135
                  tunnel: [w145] -> w132
                  tunnel: w131 -> [w145]
                  tunnel: [w144] -> w129
                  tunnel: w128 -> [w144]
                  tunnel: [w159] -> w134
                  tunnel: w138 -> [w158]
                  tunnel: w137 -> [w157]
                  tunnel: w136 -> [w156]
                  tunnel: w135 -> [w155]
                  tunnel: w132 -> [w154]
                  tunnel: w129 -> [w151]
                  tunnel: [w153] -> w123
                  tunnel: [w152] -> w119
                  tunnel: w134 -> [w162]
                  tunnel: [w161] -> w124
                  tunnel: w123 -> [w161]
                  tunnel: [w160] -> w120
                  tunnel: w119 -> [w160]
                  tunnel: cluster{u16, u16, dbl, bool} {36, 1, 0.0, TRUE} -> [w166]
                  tunnel: [w165] -> w125
                  tunnel: w124 -> [w165]
                  tunnel: [w164] -> w121
                  tunnel: w120 -> [w164]
                  tunnel: [w168] -> w126
                  tunnel: w125 -> [w168]
                  tunnel: [w167] -> w122
                  tunnel: w121 -> [w167]
                  frame #0 {
                    w142 = TRUE ("Moving")
                    n128 = Not(x=w142) -> (.not. x?=w143:bool)
                    n129 = local write "Moving"(w142) -> ()
                    n130 = local write "Stopped"(w143) -> ()
                  }
                  frame #1 {
                    n131 = local read "Movement"() -> (w150:T2)
                    n132 = Unbundle(w150) -> ("Axis"=w149:u8, "Direction(To/From)"=w148:u8, "Speed in mm/s\n (5)[0,025-20]"=w147:sgl, "IV6"=w146:bool)
                  }
                  frame #2 {
                    n133 = call <userlib>:"SubVI_Einzelschritte_IF5_IF6.vi"("VISA resource name in"=w151, "Achsen-Wahl (X)"=w158, "Geschwindigkeit\nin mm/s (5)[0,025-20]"=w156, "IF5=F/IF6=T\n(IF6=T) in"=w155, "error in"=w154, "Richtung (vEw)"=w157) -> ("VISA resource name out"=w153:refnum<visa-resource-name>, "Koordinaten IF6"=w159:T7, "error out"=w152:errorcluster)  [unwired: 3 in, 4 out]
                  }
                  frame #3 {
                    n134 = Wait (ms)(milliseconds to wait=u32 100) -> ()  [unwired: 1 out]
                    n135 = local write "Current Cordinates"(w162) -> ()
                  }
                  frame #4 {
                    n136 = local write "Movement"(w166) -> ()
                  }
                  frame #5 {
                    w171 = TRUE ("Moving")
                    n137 = Not(x=w171) -> (.not. x?=w170:bool)
                    n138 = local write "Stopped"(w171) -> ()
                    n139 = local write "Moving"(w170) -> ()
                    n140 = local write "Operation Done"("Manual movement of Platform" ("Status")) -> ()
                  }
                }
              }
              frame "Save Positions" {
                n141 = flat-sequence {
                  frame #0 {
                    n142 = local read "Current Cordinates"() -> (w178:T5)
                    n143 = local read "Position"() -> (w180:T4)
                    n144 = Unbundle(w178) -> ("X axis"=w175:sgl, "Y axis"=w176:sgl, "Z axis"=w177:sgl)  [unwired: 4 out]
                    n145 = Build Array(w175, w176, w177) -> (w179:sgl[])
                    n146 = case shown="\"Position 1\", Default" w180 {
                      tunnel: w179 -> [w181 w182 w183 w184 w185 w186 w187 w188 w189 w190]
                      frame "Position 1", Default {
                        n147 = local write "P1"(w181) -> ()
                      }
                      frame "Position 2" {
                        n148 = local write "P2"(w182) -> ()
                      }
                      frame "Position 3" {
                        n149 = local write "P3"(w183) -> ()
                      }
                      frame "Position 4" {
                        n150 = local write "P4"(w184) -> ()
                      }
                      frame "Position 5" {
                        n151 = local write "P5"(w185) -> ()
                      }
                      frame "Position 6" {
                        n152 = local write "P6"(w186) -> ()
                      }
                      frame "Position 7" {
                        n153 = local write "P7"(w187) -> ()
                      }
                      frame "Position 8" {
                        n154 = local write "P8"(w188) -> ()
                      }
                      frame "Position 9" {
                        n155 = local write "P9"(w189) -> ()
                      }
                      frame "Position 10" {
                        n156 = local write "P10"(w190) -> ()
                      }
                    }
                  }
                  frame #1 {
                    n157 = local write "Save"(FALSE ("Save Button")) -> ()
                    n158 = local write "Operation Done"("Position cordinates saved" ("Operation Done")) -> ()
                  }
                }
              }
              frame "Reset Position" {
                n159 = flat-sequence {
                  frame #0 {
                    n160 = local read "Position"() -> (w196:T4)
                    n161 = case shown="\"Position 10\"" w196 {
                      tunnel: dbl[] [0.0, 0.0, 0.0] ("P1") -> [w198 w199 w200 w201 w202 w203 w204 w205 w206 w207]
                      frame "Position 1", Default {
                        n162 = local write "P1"(w198) -> ()
                      }
                      frame "Position 2" {
                        n163 = local write "P2"(w199) -> ()
                      }
                      frame "Position 3" {
                        n164 = local write "P3"(w200) -> ()
                      }
                      frame "Position 4" {
                        n165 = local write "P4"(w201) -> ()
                      }
                      frame "Position 5" {
                        n166 = local write "P5"(w202) -> ()
                      }
                      frame "Position 6" {
                        n167 = local write "P6"(w203) -> ()
                      }
                      frame "Position 7" {
                        n168 = local write "P7"(w204) -> ()
                      }
                      frame "Position 8" {
                        n169 = local write "P8"(w205) -> ()
                      }
                      frame "Position 9" {
                        n170 = local write "P9"(w206) -> ()
                      }
                      frame "Position 10" {
                        n171 = local write "P10"(w207) -> ()
                      }
                    }
                  }
                  frame #1 {
                    n172 = local write "Reset"(FALSE ("Reset")) -> ()
                    n173 = local write "Operation Done"("The selected position is reset" ("Operation Done")) -> ()
                  }
                }
              }
              frame "Reset All" {
                n174 = flat-sequence {
                  frame #0 {
                    w213 = dbl[] [0.0, 0.0, 0.0] ("P1")
                    n175 = local write "P1"(w213) -> ()
                    n176 = local write "P2"(w213) -> ()
                    n177 = local write "P3"(w213) -> ()
                    n178 = local write "P4"(w213) -> ()
                    n179 = local write "P5"(w213) -> ()
                    n180 = local write "P6"(w213) -> ()
                    n181 = local write "P7"(w213) -> ()
                    n182 = local write "P8"(w213) -> ()
                    n183 = local write "P9"(w213) -> ()
                    n184 = local write "P10"(w213) -> ()
                    n185 = local write "Steps(mm)"(w213) -> ()
                  }
                  frame #1 {
                    n186 = local write "Reset All"(FALSE ("Reset all Positions")) -> ()
                    n187 = local write "Operation Done"("Reset all positions" ("Operation Done")) -> ()
                  }
                }
              }
              frame "Go Position" {
                n188 = flat-sequence {
                  tunnel: [w226] -> w217
                  tunnel: [w225] -> w216
                  tunnel: w221 -> [w228]
                  tunnel: w220 -> [w227]
                  tunnel: [w251] -> w218
                  tunnel: [w252] -> w219
                  tunnel: w217 -> [w252]
                  tunnel: w216 -> [w251]
                  frame #0 {
                    w224 = TRUE ("Moving")
                    n189 = local write "Moving"(w224) -> ()
                    n190 = local read "Position"() -> (w236:T4)
                    n191 = case shown="\"Position 10\"" w236 {
                      tunnel: [w237 w238 w239 w240 w241 w242 w243 w244 w245 w246] -> w234
                      frame "Position 1", Default {
                        n192 = local read "P1"() -> (w237:dbl[])
                      }
                      frame "Position 2" {
                        n193 = local read "P2"() -> (w238:dbl[])
                      }
                      frame "Position 3" {
                        n194 = local read "P3"() -> (w239:dbl[])
                      }
                      frame "Position 4" {
                        n195 = local read "P4"() -> (w240:dbl[])
                      }
                      frame "Position 5" {
                        n196 = local read "P5"() -> (w241:dbl[])
                      }
                      frame "Position 6" {
                        n197 = local read "P6"() -> (w242:dbl[])
                      }
                      frame "Position 7" {
                        n198 = local read "P7"() -> (w243:dbl[])
                      }
                      frame "Position 8" {
                        n199 = local read "P8"() -> (w244:dbl[])
                      }
                      frame "Position 9" {
                        n200 = local read "P9"() -> (w245:dbl[])
                      }
                      frame "Position 10" {
                        n201 = local read "P10"() -> (w246:dbl[])
                      }
                    }
                    n202 = Not(x=w224) -> (.not. x?=w223:bool)
                    n203 = local write "Stopped"(w223) -> ()
                    n204 = local read "Speed"() -> (w230:dbl)
                    n205 = local read "Current Cordinates"() -> (w233:T5)
                    n206 = Bundle(0, "Speed"=w230, 0) -> (w229:cluster{i32, "Speed":dbl, i32})  [unwired: 1 in]
                    n207 = call <userlib>:"SubVI_Punkt_anfahren_IF5_IF6.vi"("Angehängtes Array"=w234, "error in"=w227, "Koordinaten in IF6"=w233, "Geschwindigkeiten"=w229, "VISA resource name in"=w228) -> ("error out"=w225:errorcluster, "Koordinaten out IF6"=w235:T7, "VISA resource name in 2"=w226:refnum<visa-resource-name>)  [unwired: 1 in]
                    n208 = local write "Current Cordinates"(w235) -> ()
                  }
                  frame #1 {
                    w247 = TRUE ("Moving")
                    n209 = local write "Go To"(FALSE ("Go To")) -> ()
                    n210 = local write "Stopped"(w247) -> ()
                    n211 = Not(x=w247) -> (.not. x?=w248:bool)
                    n212 = local write "Moving"(w248) -> ()
                    n213 = local write "Operation Done"("Go to the selected position" ("Operation Done")) -> ()
                  }
                }
              }
              frame "Import Cordinates" {
                n214 = flat-sequence {
                  frame #0 {
                    n215 = local read "File Path"() -> (w266:path)
                    n216 = call "Dekoder Batch Speicher.vi"("Batchfeld Speicher"=w266) -> ("P9"=w256:dbl[], "P10"=w257:dbl[], "P1"=w258:dbl[], "P2"=w259:dbl[], "P8"=w260:dbl[], "P3"=w261:dbl[], "P4"=w262:dbl[], "P7"=w265:dbl[], "P6"=w263:dbl[], "P5"=w264:dbl[])  [unwired: 5 in]
                    n217 = local write "P9"(w256) -> ()
                    n218 = local write "P10"(w257) -> ()
                    n219 = local write "P1"(w258) -> ()
                    n220 = local write "P2"(w259) -> ()
                    n221 = local write "P8"(w260) -> ()
                    n222 = local write "P3"(w261) -> ()
                    n223 = local write "P4"(w262) -> ()
                    n224 = local write "P5"(w264) -> ()
                    n225 = local write "P6"(w263) -> ()
                    n226 = local write "P7"(w265) -> ()
                  }
                  frame #1 {
                    n227 = local write "Import"(FALSE ("Import")) -> ()
                    n228 = local write "Operation Done"("Import the position cordinates" ("Operation Done")) -> ()
                  }
                }
              }
              frame "Export Cordinates" {
                n229 = flat-sequence {
                  frame #0 {
                    n230 = Two Button Dialog(message="Copy the values to ? ", 1:"New File" ("F button name (\"Cancel\")"), 2:"Existing File" ("T button name (\"OK\")")) -> (T button?=w272:bool)
                    n231 = case shown="True" w272 {
                      frame False {
                        n232 = local read "P10"() -> (w282:dbl[])
                        n233 = local read "P1"() -> (w288:dbl[])
                        n234 = local read "P2"() -> (w287:dbl[])
                        n235 = local read "P3"() -> (w286:dbl[])
                        n236 = local read "P4"() -> (w285:dbl[])
                        n237 = local read "P5"() -> (w284:dbl[])
                        n238 = local read "P6"() -> (w283:dbl[])
                        n239 = local read "P7"() -> (w279:dbl[])
                        n240 = local read "P8"() -> (w280:dbl[])
                        n241 = local read "P9"() -> (w281:dbl[])
                        n242 = Build Array(w288, w287, w286, w285, w284, w283, w279, w280, w281, w282) -> (w276:dbl[][])
                        n243 = call-poly <vilib>:"Write To Spreadsheet File.vi"("format (%.3f)"="%.6f", "2D data"=w276) -> ("new file path (Not A Path if cancelled)"=w278:path)  [unwired: 6 in]
                        n244 = local write "File Path"(w278) -> ()
                      }
                      frame True {
                        n245 = local read "P10"() -> (w290:dbl[])
                        n246 = local read "P1"() -> (w291:dbl[])
                        n247 = local read "P2"() -> (w292:dbl[])
                        n248 = local read "P3"() -> (w293:dbl[])
                        n249 = local read "P4"() -> (w294:dbl[])
                        n250 = local read "P5"() -> (w295:dbl[])
                        n251 = local read "P6"() -> (w296:dbl[])
                        n252 = local read "P7"() -> (w297:dbl[])
                        n253 = local read "P8"() -> (w298:dbl[])
                        n254 = local read "P8"() -> (w299:dbl[])
                        n255 = Build Array(w291, w292, w293, w294, w295, w296, w297, w298, w299, w290) -> (w300:dbl[][])
                        n256 = local read "File Path"() -> (w289:path)
                        n257 = call-poly <vilib>:"Write To Spreadsheet File.vi"("format (%.3f)"="%.6f", "2D data"=w300, "file path (dialog if empty)"=w289) -> ()  [unwired: 5 in, 1 out]
                      }
                    }
                  }
                  frame #1 {
                    n258 = local write "Export"(FALSE ("Export")) -> ()
                    n259 = local write "Operation Done"("Export the position cordinates" ("Operation Done")) -> ()
                  }
                }
              }
              frame "Home Position" {
                n260 = flat-sequence {
                  tunnel: [w314] -> w311
                  tunnel: w310 -> [w314]
                  tunnel: [w313] -> w309
                  tunnel: w308 -> [w313]
                  tunnel: w311 -> [w321]
                  tunnel: w309 -> [w320]
                  tunnel: [w319] -> w306
                  tunnel: [w318] -> w304
                  tunnel: [w326] -> w307
                  tunnel: w306 -> [w326]
                  tunnel: [w325] -> w305
                  tunnel: w304 -> [w325]
                  frame #0 {
                    w315 = TRUE ("Moving")
                    n261 = Not(x=w315) -> (.not. x?=w316:bool)
                    n262 = local write "Moving"(w315) -> ()
                    n263 = local write "Stopped"(w316) -> ()
                  }
                  frame #1 {
                    w323 = u16 6 items=["X-Achse", "Y-Achse", "Z-Achse", "X- und Y-Achse", "X- und Z-Achse", "Y- und Z-Achse", "X, Y und Z-Achse", "U-Achse", "keine Achse"] ("Beteiligte Achsen (X,Y,Z,U)")
                    n264 = call "SubVI_Home_XYZU_IF5_IF6.vi"("VISA resource name in"=w320, "Beteiligte Achsen (X,Y,Z,U)"=w323, "Geschwindigkeiten"=T6 {"Geschwindigkeit X in mm/s\n(5) [0,025-15]"=10.0, "Geschwindigkeit Y in mm/s\n(5) [0,025-15]"=10.0, "Geschwindigkeit Z in mm/s\n(5) [0,025-15]"=10.0, "GeschwindigkeitU in mm/s\n(5) [0,025-15]"=2.0}, "IF5=F/IF6=T\n(IF6=T) in"=TRUE ("IF5=F/IF6=T\n(IF6=T) in"), "error in"=w321) -> ("VISA resource name out"=w319:refnum<visa-resource-name>, "Koordinaten IF6"=w322:T7, "error out"=w318:errorcluster)  [unwired: 3 in, 5 out]
                    n265 = local write "Current Cordinates"(w322) -> ()
                  }
                  frame #2 {
                    w329 = FALSE ("Moving")
                    n266 = Not(x=w329) -> (.not. x?=w330:bool)
                    n267 = local write "Moving"(w329) -> ()
                    n268 = local write "Stopped"(w330) -> ()
                    n269 = local write "Home Position"(FALSE ("Go To")) -> ()
                    n270 = local write "Operation Done"("The platform is taken to home position (0,0,0)" ("Operation Done")) -> ()
                  }
                }
              }
              frame "Load Sequence" {
                n271 = flat-sequence {
                  frame #0 {
                    n272 = local read "File  Select"() -> (w335:path)
                    n273 = call-poly <vilib>:"Read From Spreadsheet File.vi"("file path (dialog if empty)"=w335) -> ("all rows"=w334:string[][])  [unwired: 6 in, 4 out]
                    n274 = local write "Sequence"(w334) -> ()
                  }
                  frame #1 {
                    n275 = local write "Load Sequence"(FALSE ("Load Sequence")) -> ()
                    n276 = local write "Operation Done"("Sequence loaded" ("Status")) -> ()
                  }
                }
              }
              frame "Clear Sequence" {
                n277 = flat-sequence {
                  frame #0 {
                    n278 = Initialize Array("" ("element")) -> (w341:string[][])  [unwired: 2 in]
                    n279 = local write "Sequence"(w341) -> ()
                  }
                  frame #1 {
                    n280 = local write "Clear Sequence"(FALSE ("Clear Sequence")) -> ()
                    n281 = local write "Operation Done"("Sequence cleared" ("Status")) -> ()
                  }
                }
              }
              frame "Clear SensorReadings" {
                n282 = flat-sequence {
                  frame #0 {
                    n283 = local read "Clear Sensor Readings"() -> (w350:bool)
                    n284 = Initialize Array("" ("element")) -> (w351:string[][])  [unwired: 2 in]
                    n285 = local write "ED32i_output"(w351) -> ()
                    n286 = local write "ED33_output"(w351) -> ()
                    n287 = call "ED33_32i_Read.vi"("Clear"=w350) -> ()  [unwired: 5 in, 2 out]
                    n288 = property on="ED32i" class="WFChart (strict)"("History Data"=cluster{"Array 4[0]":i32, "Array 4[1]":i32}[] []) -> ()  [unwired: 2 in, 2 out]
                    n289 = property on="ED33" class="WFChart (strict)"("History Data"=i32[] []) -> ()  [unwired: 2 in, 2 out]
                  }
                  frame #1 {
                    n290 = local write "Clear Sensor Readings"(FALSE ("Clear Sensor Readings")) -> ()
                    n291 = local write "Operation Done"("Cleared sensor readings" ("Operation Done")) -> ()
                  }
                }
              }
              frame "Set Speed" {
                n292 = flat-sequence {
                  frame #0 {
                    n293 = local read "Current Sequence"() -> (w358:string[])
                    n294 = Index Array(array=w358, index=1) -> (element=w360:string)
                    n295 = Fract/Exp String To Number(string=w360) -> (number=w361:dbl)  [unwired: 3 in, 1 out]
                    n296 = local write "Speed"(w361) -> ()
                  }
                  frame #1 {
                    n297 = local write "Operation Done"("Speed Set") -> ()
                  }
                }
              }
              frame "Set Powersupply" {
                n298 = flat-sequence {
                  frame #0 {
                    n299 = local read "Current Sequence"() -> (w366:string[])
                    n300 = local read "Port for Powersupply"() -> (w372:refnum<visa-resource-name>)
                    n301 = Index Array(array=w366, index=1 ("Index")) -> (element=w368:string)
                    n302 = Concatenate Strings(w368, "\r") -> (w370:string)
                    n303 = call "Serial_com_powersupply für Funktion.vi"("VISA resource name"=w372, "write"=TRUE, "string to write"=w370) -> ()  [unwired: 6 in, 2 out]
                  }
                  frame #1 {
                    n304 = local read "Port for Write Head"() -> (w374:refnum<visa-resource-name>)
                    n305 = Concatenate Strings("GPV 6" ("string"), "\r") -> (w376:string)
                    n306 = call "Serial_com_powersupply für Funktion.vi"("VISA resource name"=w374, "write"=TRUE, "string to write"=w376) -> ()  [unwired: 6 in, 2 out]
                  }
                  frame #2 {
                    n307 = local write "Operation Done"("Powersupply Set") -> ()
                  }
                }
              }
              frame "Batch Position" {
                n308 = flat-sequence {
                  tunnel: [w387] -> w382
                  tunnel: [w386] -> w381
                  tunnel: w380 -> [w385]
                  tunnel: w379 -> [w384]
                  frame #0 {
                    n309 = local read "Current Sequence"() -> (w388:string[])
                    n310 = Index Array(array=w388, index=1) -> (element=w390:string)
                    n311 = case shown="\"Position 1\", Default" w390 {
                      tunnel: [w398 w399 w400 w401 w402 w403 w404 w405 w406 w407] -> w391
                      frame "Position 1", Default {
                        n312 = local read "P1"() -> (w398:dbl[])
                      }
                      frame "Position 2" {
                        n313 = local read "P2"() -> (w399:dbl[])
                      }
                      frame "Position 3" {
                        n314 = local read "P3"() -> (w400:dbl[])
                      }
                      frame "Position 4" {
                        n315 = local read "P4"() -> (w401:dbl[])
                      }
                      frame "Position 5" {
                        n316 = local read "P5"() -> (w402:dbl[])
                      }
                      frame "Position 6" {
                        n317 = local read "P6"() -> (w403:dbl[])
                      }
                      frame "Position 7" {
                        n318 = local read "P7"() -> (w404:dbl[])
                      }
                      frame "Position 8" {
                        n319 = local read "P8"() -> (w405:dbl[])
                      }
                      frame "Position 9" {
                        n320 = local read "P9"() -> (w406:dbl[])
                      }
                      frame "Position 10" {
                        n321 = local read "P10"() -> (w407:dbl[])
                      }
                    }
                    n322 = local read "Speed"() -> (w396:dbl)
                    n323 = Bundle(1, "Speed"=w396, 1) -> (w397:cluster{i32, "Speed":dbl, i32})  [unwired: 1 in]
                    n324 = local read "Current Cordinates"() -> (w392:T5)
                    n325 = call <userlib>:"SubVI_Punkt_anfahren_IF5_IF6.vi"("Angehängtes Array"=w391, "error in"=w385, "Koordinaten in IF6"=w392, "Geschwindigkeiten"=w397, "VISA resource name in"=w384) -> ("error out"=w386:errorcluster, "Koordinaten out IF6"=w393:T7, "VISA resource name in 2"=w387:refnum<visa-resource-name>)  [unwired: 1 in]
                    n326 = local write "Current Cordinates"(w393) -> ()
                  }
                  frame #1 {
                    n327 = local write "Operation Done"("Position Set") -> ()
                  }
                }
              }
              frame "Go Straight" {
                n328 = local read "ED32i Active?"() -> (w411:bool)
                n329 = local read "ED33 Active?"() -> (w410:bool)
                n330 = Or(x=w411, y=w410) -> (x .or. y?=w409:bool)
                n331 = case shown="False" w409 {
                  tunnel: w415 -> [w420 w452]
                  tunnel: w414 -> [w419 w455]
                  tunnel: [w418 w457] -> w413
                  tunnel: [w417 w454] -> w412
                  frame False {
                    n332 = flat-sequence {
                      tunnel: w420 -> [w434]
                      tunnel: [w436] -> w422
                      tunnel: [w435] -> w421
                      tunnel: w419 -> [w433]
                      tunnel: w422 -> [w450]
                      tunnel: [w450] -> w417
                      tunnel: [w449] -> w418
                      tunnel: w421 -> [w449]
                      frame #0 {
                        w440 = TRUE ("Moving")
                        n333 = local read "X axis"() -> (w429:enum16{"Left", "Right"})
                        n334 = local read "Y axis"() -> (w428:enum16{"Forward", "Backward"})
                        n335 = local read "Z axis"() -> (w427:enum16{"Up", "Down"})
                        n336 = case shown="\"Forward\", Default" w428 {
                          tunnel: [0 1] -> w431
                          frame "Forward", Default {
                          }
                          frame "Backward" {
                          }
                        }
                        n337 = case shown="\"Right\"" w429 {
                          tunnel: [1 0] -> w432
                          frame "Left", Default {
                          }
                          frame "Right" {
                          }
                        }
                        n338 = case shown="\"Down\"" w427 {
                          tunnel: [1 0] -> w430
                          frame "Up", Default {
                          }
                          frame "Down" {
                          }
                        }
                        n339 = local read "Steps(mm)"() -> (w426:dbl[])
                        n340 = local read "Current Sequence"() -> (w424:string[])
                        n341 = local read "Activate Sequence?"() -> (w438:bool)
                        n342 = Build Array (concatenate)(w426, w432, w431, w430) -> (w425:dbl[])
                        n343 = local read "Speed"() -> (w423:dbl)
                        n344 = Not(x=w440) -> (.not. x?=w439:bool)
                        n345 = local write "Moving"(w440) -> ()
                        n346 = local write "Stopped"(w439) -> ()
                        n347 = call "Go Straight.vi"("VISA resource name in"=w433, "Sequence Active"=w438, "array"=w424, "Speed"=w423, "Steps(mm)"=w425, "error in"=w434) -> ("VISA resource name out"=w436:refnum<visa-resource-name>, "Koordinaten IF6"=w437:T7, "error out"=w435:errorcluster)
                        n348 = local write "Current Cordinates"(w437) -> ()
                      }
                      frame #1 {
                        w451 = TRUE ("Stopped")
                        n349 = Not(x=w451) -> (.not. x?=w448:bool)
                        n350 = local write "Move Steps"(w448) -> ()
                        n351 = local write "Stopped"(w451) -> ()
                        n352 = local write "Moving"(w448) -> ()
                        n353 = local write "Operation Done"("Moved to corresponding position" ("Operation Done")) -> ()
                      }
                    }
                  }
                  frame True {
                    n354 = flat-sequence {
                      tunnel: w452 -> [w521]
                      tunnel: [w517] -> w456
                      tunnel: w455 -> [w516]
                      tunnel: [w515] -> w453
                      tunnel: [w533] -> w457
                      tunnel: w456 -> [w533]
                      tunnel: [w530] -> w454
                      tunnel: w453 -> [w530]
                      frame #0 {
                        w518 = TRUE ("Moving")
                        n355 = local read "Z axis"() -> (w512:enum16{"Up", "Down"})
                        n356 = local read "X axis"() -> (w514:enum16{"Left", "Right"})
                        n357 = local read "Y axis"() -> (w513:enum16{"Forward", "Backward"})
                        n358 = case shown="\"Backward\"" w513 {
                          tunnel: [0 1] -> w509
                          frame "Forward", Default {
                          }
                          frame "Backward" {
                          }
                        }
                        n359 = case shown="\"Right\"" w514 {
                          tunnel: [1 0] -> w510
                          frame "Left", Default {
                          }
                          frame "Right" {
                          }
                        }
                        n360 = case shown="\"Up\", Default" w512 {
                          tunnel: [1 0] -> w508
                          frame "Up", Default {
                          }
                          frame "Down" {
                          }
                        }
                        n361 = local read "Steps(mm)"() -> (w511:dbl[])
                        n362 = Build Array (concatenate)(w511, w510, w509, w508) -> (w507:dbl[])
                        n363 = local read "Activate Sequence?"() -> (w522:bool)
                        n364 = local read "Current Sequence"() -> (w523:string[])
                        n365 = call "Go Straight.vi"("VISA resource name in"=w516, "Sequence Active"=w522, "array"=w523, "Speed"=1, "Steps(mm)"=w507, "error in"=w521) -> ("VISA resource name out"=w515:refnum<visa-resource-name>, "Koordinaten IF6"=w520:T7, "error out"=w517:errorcluster)
                        n366 = Not(x=w518) -> (.not. x?=w519:bool)
                        n367 = local write "Moving"(w518) -> ()
                        n368 = local write "Current Cordinates"(w520) -> ()
                        n369 = local write "Stopped"(w519) -> ()
                      }
                      frame #1 {
                        w532 = TRUE ("Stopped")
                        n370 = Not(x=w532) -> (.not. x?=w531:bool)
                        n371 = local write "Stopped"(w532) -> ()
                        n372 = local write "Moving"(w531) -> ()
                        n373 = local write "Move Steps"(w531) -> ()
                      }
                    }
                    n374 = flat-sequence {
                      tunnel: w452 -> [w458]
                      frame #0 {
                        n375 = local read "ED32i Active?"() -> (w460:bool)
                        n376 = local read "ED33 Active?"() -> (w459:bool)
                        n377 = case shown="True" w460 {
                          selector: w460 -> [_ w462]
                          tunnel: w458 -> [_ w461]
                          frame False {
                          }
                          frame True {
                            n378 = while {
                              tunnel: w462 -> [w476]
                              tunnel: w461 -> [w475]
                              stop <- w474 stop-if-true
                              n379 = local read "Port for ED32i"() -> (w477:refnum<visa-resource-name>)
                              n380 = call "ED33_32i_Read.vi"("error in (no error)"=w475, "ED33 Active?"=FALSE, "ED32i Active?"=w476, "Port ED32i"=w477) -> ("ED32i_output"=w471:string[][])  [unwired: 2 in, 1 out]
                              n381 = local write "ED32i_output"(w471) -> ()
                              n382 = Index Array(array=w471, index (col)=0) -> (element=w470:string[])  [unwired: 1 in]
                              n383 = Index Array(array=w471, index (col)=1) -> (element=w468:string[])  [unwired: 1 in]
                              n384 = Index Array(array=w470) -> (element=w469:string)  [unwired: 1 in]
                              n385 = Index Array(array=w468) -> (element=w467:string)  [unwired: 1 in]
                              n386 = Decimal String To Number(string=w469) -> (number=w466:i32)  [unwired: 2 in, 1 out]
                              n387 = Decimal String To Number(string=w467) -> (number=w465:i32)  [unwired: 2 in, 1 out]
                              n388 = Bundle(w466, w465) -> (w464:cluster{i32, i32})  [unwired: 1 in]
                              n389 = local read "Stopped"() -> (w474:bool)
                              n390 = local write "ED32i"(w464) -> ()
                            }
                          }
                        }
                        n391 = case shown="True" w459 {
                          selector: w459 -> [_ w479]
                          tunnel: w458 -> [_ w478]
                          frame False {
                          }
                          frame True {
                            n392 = while {
                              tunnel: w479 -> [w487]
                              tunnel: w478 -> [w486]
                              stop <- w485 stop-if-true
                              n393 = local read "Port for ED33"() -> (w488:refnum<visa-resource-name>)
                              n394 = call "ED33_32i_Read.vi"("error in (no error)"=w486, "Port ED33"=w488, "ED33 Active?"=w487, "ED32i Active?"=FALSE) -> ("ED33_output"=w482:string[][])  [unwired: 2 in, 1 out]
                              n395 = local write "ED33_output"(w482) -> ()
                              n396 = Index Array(array=w482, index (col)=1) -> (element=w484:string[])  [unwired: 1 in]
                              n397 = Decimal String To Number(string=w484) -> (number=w481:i32[])  [unwired: 2 in, 1 out]
                              n398 = local read "Stopped"() -> (w485:bool)
                              n399 = local write "ED33"(w481) -> ()
                            }
                          }
                        }
                      }
                      frame #1 {
                        n400 = local read "ED32i Active?"() -> (w491:bool)
                        n401 = local read "ED33 Active?"() -> (w490:bool)
                        n402 = case shown="True" w491 {
                          selector: w491 -> [_ w495]
                          frame False {
                          }
                          frame True {
                            n403 = local read "Current Cordinates"() -> (w492:T5)
                            n404 = local read "ED32i_output"() -> (w494:string[][])
                            n405 = call "ED33_32i_Save.vi"("ED32i Active"=w495, "Cont/MM"="Continuous" ("Movement"), "ED33 Active?"=FALSE, "Current Cordinates"=w492, "ED32i_output"=w494) -> ()  [unwired: 2 in]
                          }
                        }
                        n406 = case shown="True" w490 {
                          selector: w490 -> [_ w499]
                          frame False {
                          }
                          frame True {
                            n407 = local read "Current Cordinates"() -> (w497:T5)
                            n408 = local read "ED33_output"() -> (w500:string[][])
                            n409 = call "ED33_32i_Save.vi"("ED32i Active"=FALSE, "Cont/MM"="Continuous" ("Movement"), "ED33 Active?"=w499, "Current Cordinates"=w497, "ED33_output"=w500) -> ()  [unwired: 2 in]
                          }
                        }
                        n410 = local write "Operation Done"("Read values from sensors and values saved" ("Operation Done")) -> ()
                      }
                      frame #2 {
                        w505 = FALSE ("ED32i Active?")
                        n411 = local write "ED32i Active?"(w505) -> ()
                        n412 = local write "ED33 Active?"(w505) -> ()
                        n413 = local write "Clear Sensor Readings"(TRUE ("Clear Sensor Readings")) -> ()
                        n414 = One Button Dialog(message="Sensor readings saved! ", button name ("OK")="OK") -> ()  [unwired: 1 out]
                      }
                    }
                  }
                }
              }
              frame "Set Steps" {
                n415 = flat-sequence {
                  frame #0 {
                    n416 = for {
                      N: 7 -> [_]
                      tunnel: [w557] -> w539 mode=indexing
                      i -> [w558]
                      n417 = local read "Current Sequence"() -> (w559:string[])
                      n418 = Increment(x=w558) -> (x+1=w561:i32)
                      n419 = Index Array(array=w559, index=w561) -> (element=w560:string)
                      n420 = Fract/Exp String To Number(string=w560) -> (number=w557:dbl)  [unwired: 3 in, 1 out]
                    }
                    n421 = Array To Cluster(array=w539) -> (cluster=w538:T8)
                    n422 = Unbundle(w538) -> ("[0]"=w540:dbl, "[1]"=w541:dbl, "[2]"=w542:dbl, "[3]"=w545:dbl, "[4]"=w546:dbl, "[5]"=w547:dbl)  [unwired: 3 out]
                    n423 = Bundle("[0]"=w540, "[1]"=w541, "[2]"=w542) -> (w543:cluster{"[0]":dbl, "[1]":dbl, "[2]":dbl})  [unwired: 1 in]
                    n424 = Cluster To Array(cluster=w543) -> (array=w544:dbl[])
                    n425 = case shown="1" w545 {
                      tunnel: [enum16{"Left", "Right"}."Right" enum16{"Left", "Right"}."Left"] -> w548
                      frame 0, Default {
                      }
                      frame 1 {
                      }
                    }
                    n426 = case shown="1" w546 {
                      tunnel: [enum16{"Forward", "Backward"}."Forward" enum16{"Forward", "Backward"}."Backward"] -> w550
                      frame 0, Default {
                      }
                      frame 1 {
                      }
                    }
                    n427 = case shown="1" w547 {
                      tunnel: [enum16{"Up", "Down"}."Down" enum16{"Up", "Down"}."Up"] -> w549
                      frame 0, Default {
                      }
                      frame 1 {
                      }
                    }
                    n428 = local write "Steps(mm)"(w544) -> ()
                    n429 = local write "X axis"(w548) -> ()
                    n430 = local write "Z axis"(w549) -> ()
                    n431 = local write "Y axis"(w550) -> ()
                  }
                  frame #1 {
                    n432 = local write "Operation Done"("Steps Set") -> ()
                  }
                }
              }
              frame "Set Count" {
                n433 = flat-sequence {
                  frame #0 {
                    n434 = local read "Current Sequence"() -> (w568:string[])
                    n435 = Index Array(array=w568, index=1) -> (element=w567:string)
                    n436 = Fract/Exp String To Number(string=w567) -> (number=w569:dbl)  [unwired: 3 in, 1 out]
                    n437 = local write "Count"(w569) -> ()
                  }
                  frame #1 {
                    n438 = local write "Operation Done"("Count Set") -> ()
                  }
                }
              }
              frame "Move & Measure" {
                n439 = local read "ED32i Active?"() -> (w576:bool)
                n440 = local read "ED33 Active?"() -> (w575:bool)
                n441 = Or(x=w576, y=w575) -> (x .or. y?=w571:bool)
                n442 = case shown="True" w571 {
                  tunnel: w573 -> [w578 w584]
                  tunnel: w574 -> [_ w583]
                  tunnel: [w578 w580] -> w572
                  frame False {
                  }
                  frame True {
                    n443 = local read "Count"() -> (w579:dbl)
                    n444 = for {
                      N: w579 -> [_]
                      tunnel: w584 -> [w619]
                      tunnel: w583 -> [w618]
                      tunnel: [w614] -> w581
                      w615 = TRUE
                      n445 = flat-sequence {
                        tunnel: w619 -> [w624]
                        tunnel: w618 -> [w623]
                        tunnel: [w622] -> w617
                        tunnel: [w621] -> w613
                        tunnel: w617 -> [w643]
                        tunnel: [w642] -> w614
                        tunnel: w613 -> [w642]
                        frame #0 {
                          n446 = local read "Steps(mm)"() -> (w620:dbl[])
                          n447 = local read "Y axis"() -> (w630:enum16{"Forward", "Backward"})
                          n448 = local read "Z axis"() -> (w631:enum16{"Up", "Down"})
                          n449 = local read "X axis"() -> (w632:enum16{"Left", "Right"})
                          n450 = case shown="\"Backward\"" w630 {
                            tunnel: [0 1] -> w634
                            frame "Forward", Default {
                            }
                            frame "Backward" {
                            }
                          }
                          n451 = case shown="\"Right\"" w632 {
                            tunnel: [1 0] -> w635
                            frame "Left", Default {
                            }
                            frame "Right" {
                            }
                          }
                          n452 = case shown="\"Up\", Default" w631 {
                            tunnel: [1 0] -> w633
                            frame "Up", Default {
                            }
                            frame "Down" {
                            }
                          }
                          n453 = Build Array (concatenate)(w620, w635, w634, w633) -> (w626:dbl[])
                          n454 = local read "Current Sequence"() -> (w627:string[])
                          n455 = local read "Activate Sequence?"() -> (w628:bool)
                          n456 = call "Go Straight.vi"("VISA resource name in"=w624, "Sequence Active"=w628, "array"=w627, "Speed"=1, "Steps(mm)"=w626, "error in"=w623) -> ("VISA resource name out"=w621:refnum<visa-resource-name>, "Koordinaten IF6"=w625:T7, "error out"=w622:errorcluster)
                          n457 = local write "Current Cordinates"(w625) -> ()
                        }
                        frame #1 {
                          n458 = local read "ED32i Active?"() -> (w645:bool)
                          n459 = local read "ED33 Active?"() -> (w644:bool)
                          n460 = case shown="True" w644 {
                            selector: w644 -> [_ w654]
                            tunnel: w643 -> [_ w652]
                            frame False {
                            }
                            frame True {
                              n461 = local read "Port for ED33"() -> (w653:refnum<visa-resource-name>)
                              n462 = call "ED33_32i_Read.vi"("error in (no error)"=w652, "Port ED33"=w653, "ED33 Active?"=w654, "ED32i Active?"=FALSE) -> ("ED33_output"=w649:string[][])  [unwired: 2 in, 1 out]
                              n463 = local write "ED33_output"(w649) -> ()
                              n464 = Index Array(array=w649, index (col)=1) -> (element=w651:string[])  [unwired: 1 in]
                              n465 = Decimal String To Number(string=w651, default (0L)=i64 0) -> (number=w648:i64[])  [unwired: 1 in, 1 out]
                              n466 = local write "ED33"(w648) -> ()
                            }
                          }
                          n467 = case shown="True" w645 {
                            selector: w645 -> [_ w668]
                            tunnel: w643 -> [_ w666]
                            frame False {
                            }
                            frame True {
                              n468 = local read "Port for ED32i"() -> (w667:refnum<visa-resource-name>)
                              n469 = call "ED33_32i_Read.vi"("error in (no error)"=w666, "ED33 Active?"=FALSE, "ED32i Active?"=w668, "Port ED32i"=w667) -> ("ED32i_output"=w657:string[][])  [unwired: 2 in, 1 out]
                              n470 = local write "ED32i_output"(w657) -> ()
                              n471 = Index Array(array=w657, index (col)=0) -> (element=w663:string[])  [unwired: 1 in]
                              n472 = Index Array(array=w657, index (col)=1) -> (element=w661:string[])  [unwired: 1 in]
                              n473 = Index Array(array=w663) -> (element=w662:string)  [unwired: 1 in]
                              n474 = Index Array(array=w661) -> (element=w660:string)  [unwired: 1 in]
                              n475 = Decimal String To Number(string=w662) -> (number=w659:i32)  [unwired: 2 in, 1 out]
                              n476 = Decimal String To Number(string=w660) -> (number=w658:i32)  [unwired: 2 in, 1 out]
                              n477 = Bundle(w659, w658) -> (w656:cluster{i32, i32})  [unwired: 1 in]
                              n478 = local write "ED32i"(w656) -> ()
                            }
                          }
                        }
                      }
                      n479 = local write "Current Status"("Move and measure") -> ()
                      n480 = Not(x=w615) -> (.not. x?=w616:bool)
                      n481 = local write "Moving"(w615) -> ()
                      n482 = local write "Stopped"(w616) -> ()
                    }
                    n483 = flat-sequence {
                      tunnel: [w585] -> w582
                      tunnel: w581 -> [w585]
                      tunnel: w582 -> [w609]
                      tunnel: [w609] -> w580
                      frame #0 {
                        n484 = local read "ED32i Active?"() -> (w587:bool)
                        n485 = local read "ED33 Active?"() -> (w586:bool)
                        n486 = case shown="True" w586 {
                          selector: w586 -> [_ w595]
                          frame False {
                          }
                          frame True {
                            n487 = local read "Steps(mm)"() -> (w589:dbl[])
                            n488 = local read "Current Cordinates"() -> (w591:T5)
                            n489 = local read "ED33_output"() -> (w593:string[][])
                            n490 = Index Array(array=w589, index=1) -> (element=w588:dbl)
                            n491 = call "ED33_32i_Save.vi"("Min_move"=w588, "ED32i Active"=FALSE, "Cont/MM"="Move&Measure" ("Movement"), "ED33 Active?"=w595, "Current Cordinates"=w591, "ED33_output"=w593) -> ()  [unwired: 1 in]
                          }
                        }
                        n492 = case shown="True" w587 {
                          selector: w587 -> [_ w603]
                          frame False {
                          }
                          frame True {
                            n493 = local read "Steps(mm)"() -> (w598:dbl[])
                            n494 = local read "Current Cordinates"() -> (w599:T5)
                            n495 = local read "ED32i_output"() -> (w601:string[][])
                            n496 = Index Array(array=w598, index=1) -> (element=w596:dbl)
                            n497 = call "ED33_32i_Save.vi"("Min_move"=w596, "ED32i Active"=w603, "Cont/MM"="Move&Measure" ("Movement"), "ED33 Active?"=FALSE, "Current Cordinates"=w599, "ED32i_output"=w601) -> ()  [unwired: 1 in]
                          }
                        }
                      }
                      frame #1 {
                        w611 = TRUE
                        w608 = FALSE
                        n498 = local write "Clear Sensor Readings"(TRUE ("Clear Sensor Readings")) -> ()
                        n499 = local write "Move & Measure"(w608) -> ()
                        n500 = Not(x=w611) -> (.not. x?=w610:bool)
                        n501 = local write "Stopped"(w611) -> ()
                        n502 = local write "ED33 Active?"(w608) -> ()
                        n503 = local write "ED32i Active?"(w608) -> ()
                        n504 = local write "Operation Done"("Moved and Measured") -> ()
                        n505 = One Button Dialog(message="Sensor readings saved! ", button name ("OK")="OK") -> ()  [unwired: 1 out]
                        n506 = local write "Moving"(w610) -> ()
                      }
                    }
                  }
                }
              }
              frame "Read Sensors" {
                n507 = flat-sequence {
                  frame #0 {
                    n508 = local read "Current Sequence"() -> (w674:string[])
                    n509 = Index Array(array=w674, index=1) -> (element=w672:string)
                    n510 = case shown="\"ED33\"" w672 {
                      frame "ED32i", Default {
                        n511 = local write "ED32i Active?"(TRUE ("ED32i Active?")) -> ()
                      }
                      frame "ED33" {
                        n512 = local write "ED33 Active?"(TRUE ("ED33 Active?")) -> ()
                      }
                    }
                  }
                  frame #1 {
                    n513 = local write "Operation Done"("Sensor selected") -> ()
                  }
                }
              }
              frame "Write Pole" {
                n514 = local read "Port for Powersupply"() -> (w681:refnum<visa-resource-name>)
                n515 = local read "Current Sequence"() -> (w683:string[])
                n516 = local read "Port for Write Head"() -> (w682:refnum<visa-resource-name>)
                n517 = call "Write Pole.vi"("Fehler (Eingang)"=w680, "array"=w683, "Port for write head"=w682, "Port for Powersupply"=w681) -> ("Fehler (Ausgang)"=w679:errorcluster)
              }
            }
          }
          frame Error {
            n518 = Unbundle(w686) -> ("source"=w685:string)  [unwired: 2 out]
            n519 = One Button Dialog(message=w685) -> (true=w689:bool)  [unwired: 1 in]
            n520 = local write "Stop Program"(w689) -> ()
            n521 = local write "Stopped"(w689) -> ()
            n522 = local write "Current Status"("Force stop due to error" ("Status")) -> ()
          }
        }
        n523 = local read "Stop Program"() -> (w38:bool)
        n524 = flat-sequence {
          tunnel: [w66] -> w45
          tunnel: w46 -> [w65]
          frame #0 {
            n525 = local read "Current Status"() -> (w67:string)
            n526 = case shown="\"Waiting for next instruction\"" w67 {
              selector: w67 -> [w69 _]
              tunnel: [w69 w70] -> w66
              tunnel: w65 -> [_ w70]
              frame "Pause", Default {
                n527 = local write "Current Status"("Waiting for next instruction" ("Status")) -> ()
              }
              frame "Waiting for next instruction" {
              }
            }
          }
        }
        n528 = case shown="True" w38 {
          frame False {
          }
          frame True {
            w62 = FALSE ("Moving")
            n529 = local write "Moving"(w62) -> ()
            n530 = Not(x=w62) -> (.not. x?=w63:bool)
            n531 = local write "Stopped"(w63) -> ()
            n532 = local write "Operation Done"("Program Stopped!!!" ("Status")) -> ()
          }
        }
      }
    }
  }
  n533 = local write "Error Out"(w1) -> ()
  n534 = call <vilib>:"General Error Handler.vi"("error in (no error)"=w1) -> ()  [unwired: 10 in, 5 out]
